vi "Tuning.vi"() -> ()   [LabVIEW 2018]
uses:
  Type/_GUI Method.ctl
  Type/_Lens Property.ctl
  Type/_Mass Range Property.ctl
  Type/_Mass Range Parameters.ctl
  Type/_RT Res Type.ctl
  Type/_Run Mode.ctl
  Type/_Run State.ctl
  Type/_File Type.ctl
  Type/_RT Command.ctl
  Type/_Data Operation.ctl
  Type/_Run Module.ctl
  Configuration/_Global Configuration.vi
  <vilib>/Utility/config.llb/Read Key (Path).vi
  <vilib>/Utility/config.llb/Read Key (Boolean).vi
  <vilib>/Utility/config.llb/Read Key (String).vi
  <vilib>/printing/ReportDocExtensions.llb/Append Front Panel Image to Report (path).vi
  <vilib>/Utility/config.llb/Write Key (Path).vi
  <vilib>/Utility/config.llb/Write Key (Boolean).vi
  <vilib>/Utility/config.llb/Write Key (String).vi
  <vilib>/Utility/miscctls.llb/LVRectTypeDef.ctl
  Type/_PIC Channel.ctl
  <vilib>/Utility/NIReport.llb/NI_report.lvclass
  <vilib>/Utility/NIReport.llb/NI_ReportGenerationCore.lvlib
  <vilib>/Utility/config.llb/NI_LVConfig.lvlib
panel:
  in  "Run 2":bool
  in  "Cancel":bool
  in  "NewMethod":bool
  in  "Method Path":path=path "C:/Users/Min/Projects/Sniffer/Build/Tune Method.d2m"
  in  "Tab":T1(tab)=enum."Mass Ranges"
  in  "Export Settings":bool
  out "Use Pol Swap Options from Config":bool
  in  "Delay Time (ms)":dbl=1.0 format="%#.3f"
  in  "CEM POL":bool
  in  "Polarity":enum32{"Positive Ions", "Negative Ions"}(radio) caption="Cal/Res Table Select"
  in  "Count1":dbl=420.0 caption="User Value" format="%.3f"
  in  "Q1DC POL":bool
  in  "Q2DC POL":bool
  out "DAC Value":i32=6174
  in  "Parameter Table":i32(listbox)
  in  "Swtich Polarity":bool
  in  "Ramping Parameter":u8(ring)=7 items=["Q1 RF", "Q1 DC", "Q1 RR", "Q2 RF", "Q2 DC", "Q2 RR", "M1 RF", "EV", "ED", "MO", "RO L1", "M1", "RO L2", "M2", "RO L3", "RO PF", "Q1", "CC L1", "CC L2", "CC", "CC L3", "CC L4", "Q2", "DD", "DISC", "DV", "DET horn", "HED", "EL", "LS400A", "LS-400A", "LS400B", "LS-400B", "QPS800", "QPS-800", "DG", "NG1", "HG1", "NG2", "HG2", "CC P", "SX", "ISV2", "ISV1", "CD", "CAP"]
  in  "Step Value":dbl=5.0 format="%#.3f"
  in  "Stop Value":dbl=80.0 format="%#.3f"
  in  "Start Value":dbl=10.0 format="%#.3f"
  in  "Perform Parameter Ramp":bool
  in  "Center/Width":bool
  in  "Scan Parameter with Mass":bool
  out "# of Steps":i32=141
  in  "Fixed Mass (amu)":dbl min=0.0
  in  "Scan Type":T2=enum."Q1 Scan"
  in  "Run Duration (s)":dbl=0.707 format="%#.3f"
  out "Cycle Time (ms)":dbl=706.0 format="%#.3f"
  in  "# of Cycles":i32=1
  in  "Pause Time (ms)":dbl=1.0 format="%#.3f"
  in  "Insert Row":bool
  in  "Delete Row":bool
  out "Ramp Time (ms)":dbl=705.0 format="%#.3f"
  in  "Dwell Time (ms)":dbl=5.0 min=0.001 format="%#.3f"
  in  "Step Mass (amu)":dbl=0.1 format="%#.3f"
  in  "Stop Mass (amu)":dbl=614.0 min=0.0 format="%#.3f"
  in  "Mass Range":i32(listbox)
  in  "Start Mass (amu)":dbl=600.0 min=0.0 format="%#.3f"
  in  "MR Parameters":bool
  in  "Resolution (Q1/Q2)":T3=2 items=["High/High", "Medium/Medium", "Low/Low", "High/Medium", "High/Low", "Medium/High", "Medium/Low", "Low/High", "Low/Medium"]
  in  "Method":T4={"Lenses"=[{"Scan Type"=0, "Scans"=1, "Time 1"=1.0, "Time 2"=1.0, "Value 1"=400.0, "Value 2"=400.0, "Step Size"=1.0}, {"Scan Type"=0, "Scans"=1, "Time 1"=1.0, "Time 2"=1.0, "Value 1"=150.0, "Value 2"=150.0, "Step Size"=1.0}, {"Scan Type"=0, "Scans"=1, "Time 1"=1.0, "Time 2"=1.0, "Value 1"=32000.0, "Value 2"=32000.0, "Step Size"=1.0}, {"Scan Type"=0, "Scans"=1, "Time 1"=1.0, "Time 2"=1.0, "Value 1"=400.0, "Value 2"=400.0, "Step Size"=1.0}, {"Scan Type"=0, "Scans"=1, "Time 1"=1.0, "Time 2"=1.0, "Value 1"=150.0, "Value 2"=150.0, "Step Size"=1.0}, {"Scan Type"=0, "Scans"=1, "Time 1"=1.0, "Time 2"=1.0, "Value 1"=64000.0, "Value 2"=64000.0, "Step Size"=1.0}, {"Scan Type"=0, "Scans"=1, "Time 1"=1.0, "Time 2"=1.0, "Value 1"=420.0, "Value 2"=420.0, "Step Size"=1.0}, {"Scan Type"=0, "Scans"=1, "Time 1"=1.0, "Time 2"=1.0, "Value 1"=30.0, "Value 2"=30.0, "Step Size"=1.0}, {"Scan Type"=0, "Scans"=1, "Time 1"=1.0, "Time 2"=1.0, "Value 1"=15.0, "Value 2"=15.0, "Step Size"=1.0}, {"Scan Type"=0, "Scans"=1, "Time 1"=1.0, "Time 2"=1.0, "Value 1"=0.0, "Value 2"=0.0, "Step Size"=1.0}, {"Scan Type"=0, "Scans"=1, "Time 1"=1.0, "Time 2"=1.0, "Value 1"=0.0, "Value 2"=0.0, "Step Size"=1.0}, {"Scan Type"=0, "Scans"=1, "Time 1"=1.0, "Time 2"=1.0, "Value 1"=0.0, "Value 2"=0.0, "Step Size"=1.0}, {"Scan Type"=0, "Scans"=1, "Time 1"=1.0, "Time 2"=1.0, "Value 1"=0.0, "Value 2"=0.0, "Step Size"=1.0}, {"Scan Type"=0, "Scans"=1, "Time 1"=1.0, "Time 2"=1.0, "Value 1"=0.0, "Value 2"=0.0, "Step Size"=1.0}, {"Scan Type"=0, "Scans"=1, "Time 1"=1.0, "Time 2"=1.0, "Value 1"=-0.5, "Value 2"=-0.5, "Step Size"=1.0}, {"Scan Type"=0, "Scans"=1, "Time 1"=1.0, "Time 2"=1.0, "Value 1"=-2.0, "Value 2"=-2.0, "Step Size"=1.0}, {"Scan Type"=0, "Scans"=1, "Time 1"=1.0, "Time 2"=1.0, "Value 1"=-1.2, "Value 2"=-1.2, "Step Size"=1.0}, {"Scan Type"=0, "Scans"=1, "Time 1"=1.0, "Time 2"=1.0, "Value 1"=0.0, "Value 2"=0.0, "Step Size"=1.0}, {"Scan Type"=0, "Scans"=1, "Time 1"=1.0, "Time 2"=1.0, "Value 1"=-240.0, "Value 2"=-240.0, "Step Size"=1.0}, {"Scan Type"=0, "Scans"=1, "Time 1"=1.0, "Time 2"=1.0, "Value 1"=-50.0, "Value 2"=-50.0, "Step Size"=1.0}, {"Scan Type"=0, "Scans"=1, "Time 1"=1.0, "Time 2"=1.0, "Value 1"=-52.0, "Value 2"=-52.0, "Step Size"=1.0}, {"Scan Type"=0, "Scans"=1, "Time 1"=1.0, "Time 2"=1.0, "Value 1"=-100.0, "Value 2"=-100.0, "Step Size"=1.0}, {"Scan Type"=0, "Scans"=1, "Time 1"=1.0, "Time 2"=1.0, "Value 1"=-54.0, "Value 2"=-54.0, "Step Size"=1.0}, {"Scan Type"=0, "Scans"=1, "Time 1"=1.0, "Time 2"=1.0, "Value 1"=-400.0, "Value 2"=-400.0, "Step Size"=1.0}, {"Scan Type"=0, "Scans"=1, "Time 1"=1.0, "Time 2"=1.0, "Value 1"=30.0, "Value 2"=30.0, "Step Size"=1.0}, {"Scan Type"=0, "Scans"=1, "Time 1"=1.0, "Time 2"=1.0, "Value 1"=2000.0, "Value 2"=2000.0, "Step Size"=1.0}, {"Scan Type"=0, "Scans"=1, "Time 1"=1.0, "Time 2"=1.0, "Value 1"=-6000.0, "Value 2"=-6000.0, "Step Size"=1.0}, {"Scan Type"=0, "Scans"=1, "Time 1"=1.0, "Time 2"=1.0, "Value 1"=0.0, "Value 2"=0.0, "Step Size"=1.0}, {"Scan Type"=0, "Scans"=1, "Time 1"=1.0, "Time 2"=1.0, "Value 1"=0.0, "Value 2"=0.0, "Step Size"=1.0}, {"Scan Type"=0, "Scans"=1, "Time 1"=1.0, "Time 2"=1.0, "Value 1"=250.0, "Value 2"=250.0, "Step Size"=1.0}, {"Scan Type"=0, "Scans"=1, "Time 1"=1.0, "Time 2"=1.0, "Value 1"=-250.0, "Value 2"=-250.0, "Step Size"=1.0}, {"Scan Type"=0, "Scans"=1, "Time 1"=1.0, "Time 2"=1.0, "Value 1"=250.0, "Value 2"=250.0, "Step Size"=1.0}, {"Scan Type"=0, "Scans"=1, "Time 1"=1.0, "Time 2"=1.0, "Value 1"=-250.0, "Value 2"=-250.0, "Step Size"=1.0}, {"Scan Type"=0, "Scans"=1, "Time 1"=1.0, "Time 2"=1.0, "Value 1"=500.0, "Value 2"=500.0, "Step Size"=1.0}, {"Scan Type"=0, "Scans"=1, "Time 1"=1.0, "Time 2"=1.0, "Value 1"=-500.0, "Value 2"=-500.0, "Step Size"=1.0}, {"Scan Type"=0, "Scans"=1, "Time 1"=1.0, "Time 2"=1.0, "Value 1"=0.55, "Value 2"=0.55, "Step Size"=1.0}, {"Scan Type"=0, "Scans"=1, "Time 1"=1.0, "Time 2"=1.0, "Value 1"=0.0, "Value 2"=0.0, "Step Size"=1.0}, {"Scan Type"=0, "Scans"=1, "Time 1"=1.0, "Time 2"=1.0, "Value 1"=100.0, "Value 2"=100.0, "Step Size"=1.0}, {"Scan Type"=0, "Scans"=1, "Time 1"=1.0, "Time 2"=1.0, "Value 1"=0.0, "Value 2"=0.0, "Step Size"=1.0}, {"Scan Type"=0, "Scans"=1, "Time 1"=1.0, "Time 2"=1.0, "Value 1"=5.0, "Value 2"=5.0, "Step Size"=1.0}, {"Scan Type"=0, "Scans"=1, "Time 1"=1.0, "Time 2"=1.0, "Value 1"=0.0, "Value 2"=0.0, "Step Size"=1.0}, {"Scan Type"=0, "Scans"=1, "Time 1"=1.0, "Time 2"=1.0, "Value 1"=0.0, "Value 2"=0.0, "Step Size"=1.0}, {"Scan Type"=0, "Scans"=1, "Time 1"=1.0, "Time 2"=1.0, "Value 1"=100.0, "Value 2"=100.0, "Step Size"=1.0}, {"Scan Type"=0, "Scans"=1, "Time 1"=1.0, "Time 2"=1.0, "Value 1"=0.0, "Value 2"=0.0, "Step Size"=1.0}, {"Scan Type"=0, "Scans"=1, "Time 1"=1.0, "Time 2"=1.0, "Value 1"=5.0, "Value 2"=5.0, "Step Size"=1.0}, {"Scan Type"=0, "Scans"=1, "Time 1"=1.0, "Time 2"=1.0, "Value 1"=5000.0, "Value 2"=5000.0, "Step Size"=1.0}, {"Scan Type"=0, "Scans"=1, "Time 1"=1.0, "Time 2"=1.0, "Value 1"=0.0, "Value 2"=0.0, "Step Size"=1.0}, {"Scan Type"=0, "Scans"=1, "Time 1"=1.0, "Time 2"=1.0, "Value 1"=100.0, "Value 2"=100.0, "Step Size"=1.0}, {"Scan Type"=0, "Scans"=1, "Time 1"=1.0, "Time 2"=1.0, "Value 1"=0.0, "Value 2"=0.0, "Step Size"=1.0}, {"Scan Type"=0, "Scans"=1, "Time 1"=1.0, "Time 2"=1.0, "Value 1"=5.0, "Value 2"=5.0, "Step Size"=1.0}, {"Scan Type"=0, "Scans"=1, "Time 1"=1.0, "Time 2"=1.0, "Value 1"=1000.0, "Value 2"=1000.0, "Step Size"=1.0}, {"Scan Type"=0, "Scans"=1, "Time 1"=1.0, "Time 2"=1.0, "Value 1"=1.0, "Value 2"=1.0, "Step Size"=1.0}], "Mass Ranges"=[{"Start"=600.0, "Stop"=614.0, "Step Size"=0.1, "Steps"=141, "Dwell"=5.0, "Parameters"=[], "Res"=2}], "Acquire"=FALSE, "MCA"=FALSE, "Q1DC EN"=FALSE, "Q1 POL"=FALSE, "Q3 POL"=FALSE, "Q1 RF  EN"=TRUE, "Averaging"=FALSE, "Log Scale"=FALSE, "CPS"=TRUE, "Unit"=FALSE, "Data Path"=path "C:/Users/Min/Projects/Sniffer/Build/My Data.isd", "Run Mode"=enum."Q1 Scan", "Fixed Mass (amu)"=0.0, "Q3DC EN"=FALSE, "Q3 RF  EN"=TRUE, "Negative"=FALSE} {"Mass Ranges"."Res" items=["High/High", "Medium/Medium", "Low/Low", "High/Medium", "High/Low", "Medium/High", "Medium/Low", "Low/High", "Low/Medium"]}
  out "Run Time":i32 caption="Run Time (ms)"
  in  "Log Scale":bool
  in  "Scan#":u32 caption="Current Scan #"
  in  "CPS":bool=TRUE
  in  "Averaging":bool
  in  "MCA":bool
  in  "Acquire":bool
  out "Spectrum":cluster{"Mass":dbl[], "Data in cps":dbl[]}[](graph)=[{"Mass"=[664.0], "Data in cps"=[]}, {"Mass"=[800.0], "Data in cps"=[]}, {"Mass"=[700.0], "Data in cps"=[]}]
  in  "BloUpdate":bool
  out "Data File:":path=path "C:/Users/Min/Projects/Sniffer/Build/My Data.isd"
  # "Selected Parameter Value"
  # "Selected Mass Range"
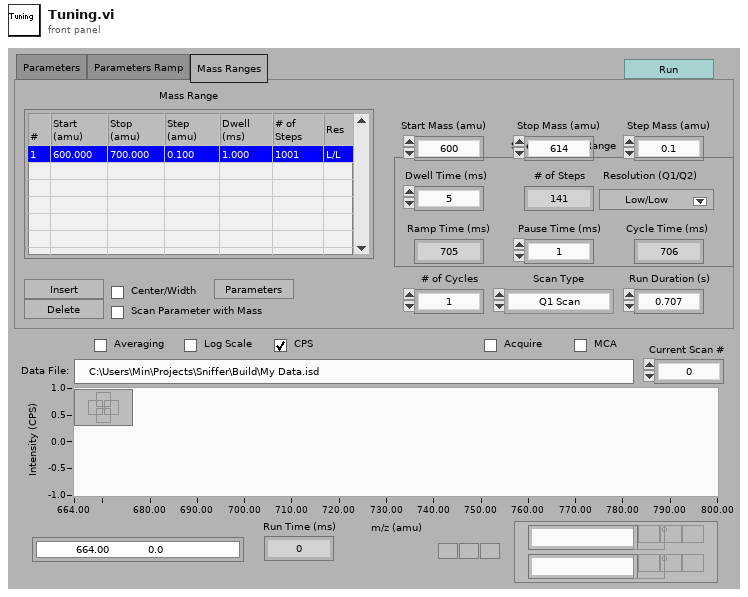
[diagram p1: front panel]
types:
  T1 = enum32{"Parameters", "Parameters Ramp", "Mass Ranges"}
  T2 = typedef "_Run Mode.ctl" = enum16{"MRM (Q1/Q2)", "Q1 Scan", "Q1 SRM", "Q2 Scan", "Q2 SRM", "Product Scan", "Precursor Scan", "Neutral Loss", "Neutral Gain"}
  T3 = typedef "_RT Res Type.ctl" = u16
  T4 = typedef "_GUI Method.ctl" = cluster{"Lenses":T5[], "Mass Ranges":T6[], "Acquire":bool, "MCA":bool, "Q1DC EN":bool, "Q1 POL":bool, "Q3 POL":bool, "Q1 RF  EN":bool, "Averaging":bool, "Log Scale":bool, "CPS":bool, "Unit":bool, "Data Path":path, "Run Mode":T2, "Fixed Mass (amu)":dbl, "Q3DC EN":bool, "Q3 RF  EN":bool, "Negative":bool}
  T5 = typedef "_Lens Property.ctl" = cluster{"Scan Type":u8, "Scans":i32, "Time 1":dbl, "Time 2":dbl, "Value 1":dbl, "Value 2":dbl, "Step Size":dbl}
  T6 = typedef "_Mass Range Property.ctl" = cluster{"Start":dbl, "Stop":dbl, "Step Size":dbl, "Steps":i32, "Dwell":dbl, "Parameters":T7[], "Res":T3}
  T7 = typedef "_Mass Range Parameters.ctl" = cluster{"Name":string, "Ch#":u8, "StartV":dbl, "StopV":dbl, "StepV":dbl, "Index":u8}
  T8 = typedef "_Run State.ctl" = enum16{"Init", "Update", "Start", "End", "Error"}
  T9 = typedef "_File Type.ctl" = enum16{"Configuration", "Old Configuration", "Calibration", "Resolution", "Diagnostic Method", "Old Method", "Acq Method", "Samp List"}
  T10 = typedef "LVRectTypeDef.ctl" = cluster{"Left":i16, "Top":i16, "Right":i16, "Bottom":i16}
  T11 = enum16{"Standard Report", "HTML", "Word", "Excel"}
  T12 = typedef "_RT Command.ctl" = enum16{"xml Start Run", "xml Start Actual Run", "xml Stop Run", "xml Runtime Update", "xml Get Status", "xml Get Table", "xml Set Table", "xml Get Configuration", "xml System Status", "xml Set LC Input Logic", "xml Get Data", "xml Get Info", "Start", "StartActualRun", "Stop", "Runtime Update", "Get Data", "Get Info", "Get Status", "Get Param", "Get Config", "Get Table", "Read ADC", "Set Oscillator", "Update Config", "Update Table", "Set All Pol", "Set Pol and DC", "Set Max Mass", "Toggle RP", "Toggle EL", "Set PIC", "Initialize Turbo", "Send Turbo Comm", "Close Turbo", "P1", "P2", "P3", "Send Serial", "Set LC Out", "Get LC In", "Read VAC", "Test Table", "Toggle Power", "Get Startup", "Set Startup", "Get ADC Table", "Set ADC Table", "Get Brief Status", "Get Detail Status", "Auxiliary Update", "Set CC Logics", "Set CC Input Logics", "Ignore Error", "invalid"}
  T13 = typedef "_Data Operation.ctl" = enum8{"Initialize", "Get Data", "Set Data", "Close"}
  T14 = enum32{"Bad", "Idle", "Run top level", "Running"}
  T15 = enum32{"existing file", "new file", "new or existing file", "existing dir", "new dir", "new or existing dir", "existing file (use LLBs)", "new file (use LLBs)", "new or existing file (use LLBs)", "new or existing file or directory (use LLBs)"}
  T16 = typedef "_PIC Channel.ctl" = enum16{"Corona +HV", "Corona -HV", "HSID Temp", "Time Const 1", "Curtain Cap +HV", "Curtain Cap -HV", "Time Const 2", "Source 1 +HV", "Source 1 -HV", "Source 1 Temp", "Time Const 3", "Source 2 +HV", "Source 2 -HV", "Source 2 Temp", "Time Const 4"}
  T17 = typedef "NI_LVConfig.lvlib/Config Data RefNum.ctl" = refnum<k1>
  T18 = typedef "_RT Instrument 2.ctl" = cluster{"Table":T19[], "Instrument":string[]}
  T19 = typedef "_RT Configuration 2.ctl" = cluster{"Name":string, "Ch#":u8, "Min":dbl, "Max":dbl, "Def+":dbl, "Def-":dbl, "Offset":dbl, "Slope":dbl, "Type":u8, "Description":string, "SettleT":dbl}
  T20 = cluster{"Method":T4, "Update":bool, "Running":bool, "Method Path":path, "BlockUpdate":bool}
  T21 = typedef "_Current Data.ctl" = cluster{"Scan#":i32, "Run Time (mS)":i32, "TIC X":dbl[], "TIC Y":dbl[][], "MassRange":cluster{"X Title":string, "X":dbl[], "Y":i32[]}[], "Fixed Mass (amu)":dbl, "Method":T22}
  T22 = typedef "_XML Expt.ctl" = cluster{"StartT(mS)":i32, "#Cycles":i32, "PauseT(uS)":i32, "ScanType":i32, "Polarity":u8, "FixedMass":dbl, "DelayT(mS)":i32, "Active Ch":T23[], "Mass Range":T6[]}
  T23 = typedef "_XML Lens.ctl" = cluster{"Value":dbl, "ChID":u8}
  T24 = typedef "_Run Module.ctl" = u16
  T25 = cluster{"Lenses":T5[], "Mass Ranges":T6[], "Acquire":bool, "MCA":bool, "Q1DC EN":bool, "Q1 POL":bool, "Q3 POL":bool, "Q1 RF  EN":bool, "Averaging":bool, "Log Scale":bool, "CPS":bool, "Unit":bool, "Data Path":path, "Run Mode":T2, "Fixed Mass (amu)":dbl, "Q3DC EN":bool, "Q3 RF  EN":bool, "Negative":bool}
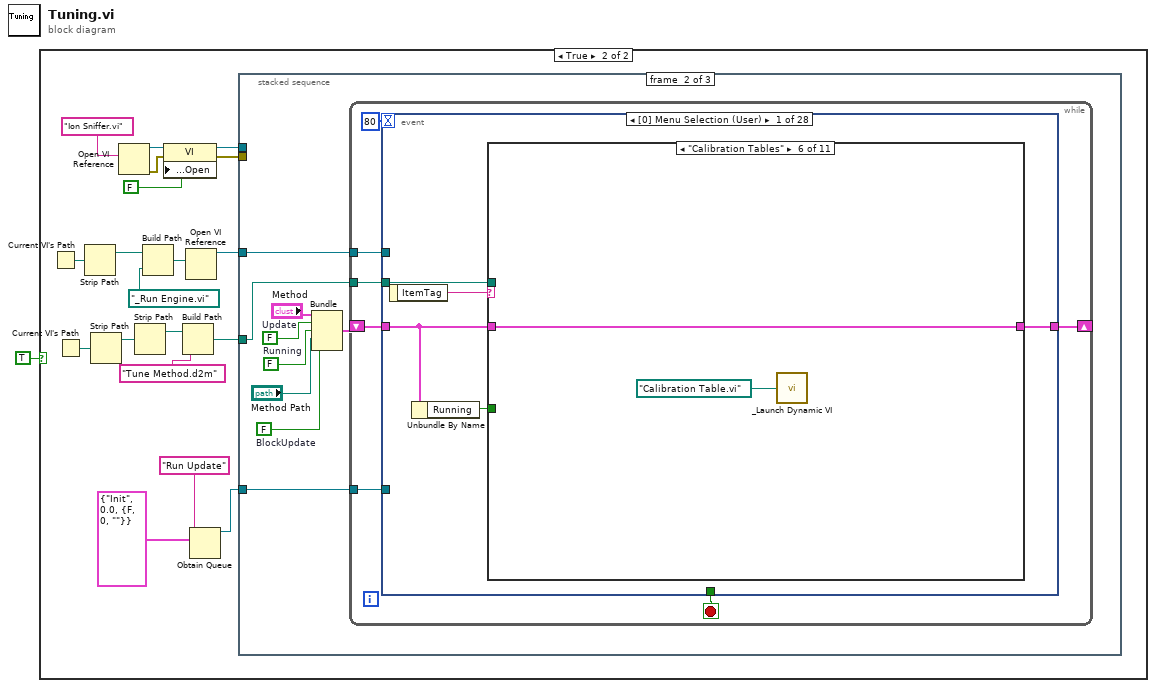
[diagram p0: block diagram]
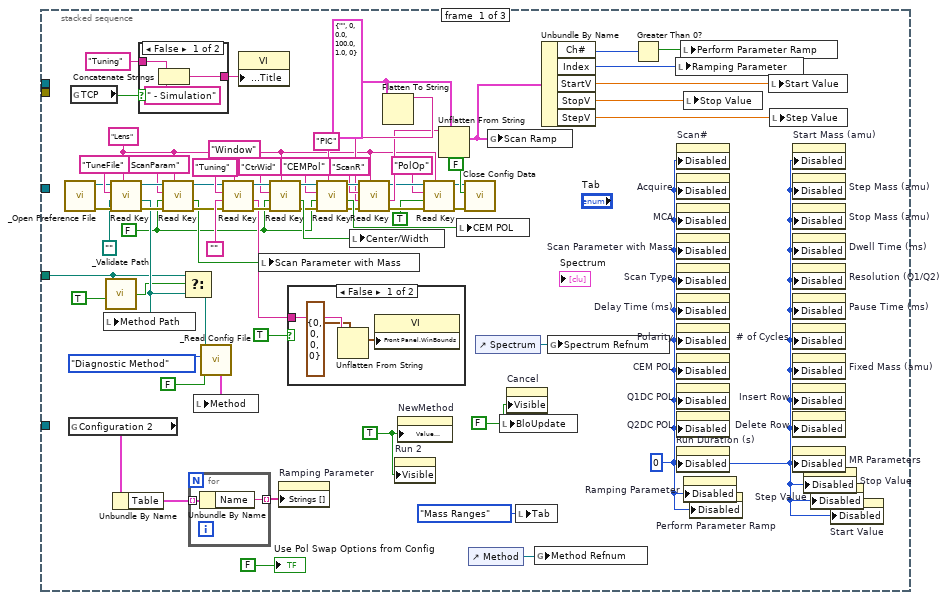
[diagram p3: hidden frame]
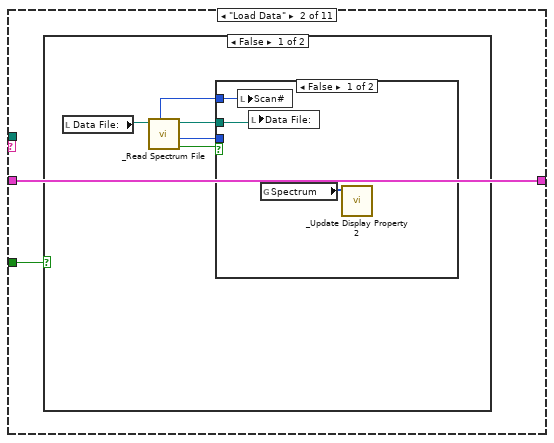
[diagram p7: hidden frame]
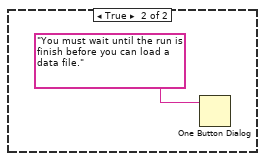
[diagram p9: hidden frame]
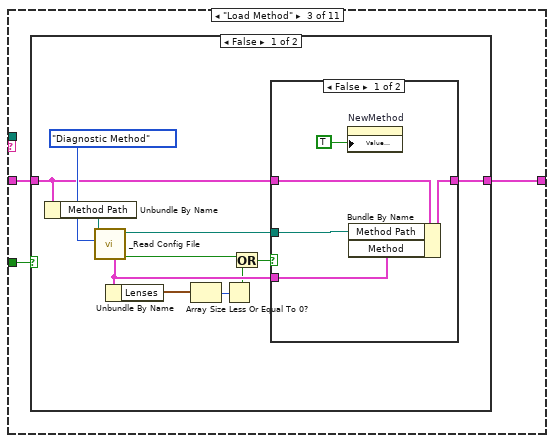
[diagram p10: hidden frame]
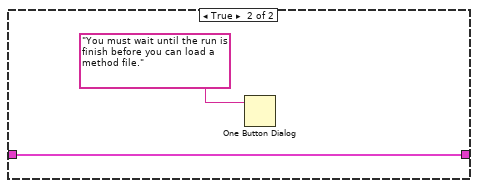
[diagram p12: hidden frame]
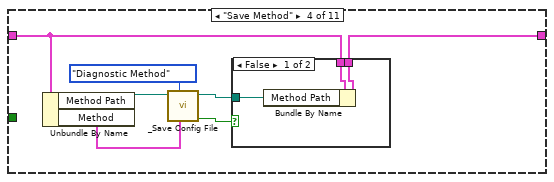
[diagram p13: hidden frame]
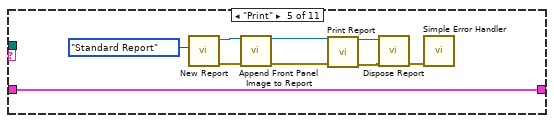
[diagram p15: hidden frame]
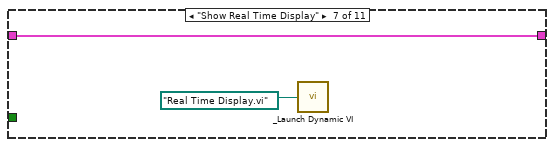
[diagram p16: hidden frame]
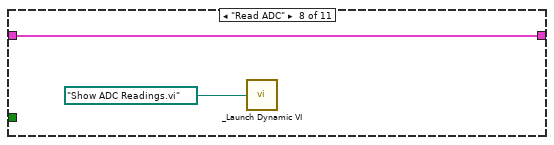
[diagram p17: hidden frame]
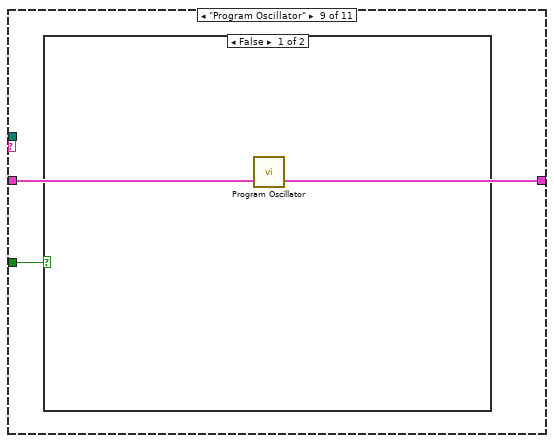
[diagram p18: hidden frame]
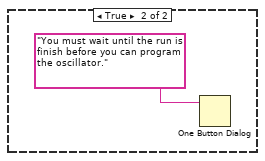
[diagram p19: hidden frame]
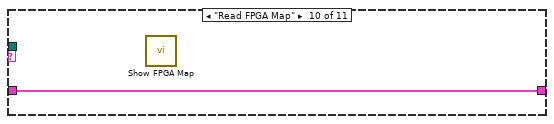
[diagram p20: hidden frame]
diagram:
  n1 = case shown="True" TRUE {
    frame False {
    }
    frame True {
      n2 = Current VI's Path() -> (path=w17:path)
      n3 = Current VI's Path() -> (path=w9:path)
      n4 = Strip Path(path=w17) -> (stripped path=w13:path)  [unwired: 1 out]
      n5 = Strip Path(path=w9) -> (stripped path=w10:path)  [unwired: 1 out]
      n6 = Open VI Reference(vi path="Ion Sniffer.vi") -> (vi reference=w5:refnum<vi>, error out=w6:errorcluster)  [unwired: 1 in, 4 out]
      n7 = Strip Path(path=w10) -> (stripped path=w11:path)  [unwired: 1 out]
      n8 = Build Path(base path=w13, name or relative path=path "_Run Engine.vi") -> (appended path=w15:path)
      n9 = property class="VI"(reference=w5, error in=w6, "Front Panel Window:Open"=FALSE) -> (reference out=w3:refnum<vi>, error out=w2:errorcluster)
      n10 = Build Path(base path=w11, name or relative path="Tune Method.d2m") -> (appended path=w8:path)
      n11 = Open VI Reference(vi path=w15) -> (vi reference=w14:refnum<vi>)  [unwired: 1 in, 5 out]
      n12 = Obtain Queue(name (unnamed)="Run Update", element data type=cluster{T8, dbl, "error out":errorcluster} {enum."Init", 0.0, "error out"={"status"=FALSE, "code"=0, "source"=""}}) -> (queue out=w18:refnum<queue>)  [unwired: 3 in, 2 out]
      n13 = stacked-sequence {
        tunnel: w18 -> [_ w105 w843]
        tunnel: w14 -> [_ w104 w842]
        tunnel: w8 -> [w50 w98 _]
        tunnel: w3 -> [_ _ w838]
        tunnel: w2 -> [_ _ w837]
        frame #0 {
          w42 = T7 {"Name"="", "Ch#"=0, "StartV"=0.0, "StopV"=100.0, "StepV"=1.0, "Index"=0} ("MR Parameters")
          w30 = u8 0 ("Disabled")
          w53 = FALSE
          w25 = "Lens" ("section")
          w71 = TRUE ("Visible")
          w79 = FALSE ("Unit")
          n14 = call "_Open Preference File.vi"() -> ("error"=w81:errorcluster, "refnum"=w82:T17)  [unwired: 3 in, 3 out]
          n15 = global read "_Global Configuration.vi" "Configuration 2"() -> (w35:T18)
          n16 = global read "_Global Configuration.vi" "TCP"() -> (w85:bool)
          n17 = call "_Validate Path.vi"("Check Exist (F)"=TRUE, "path"=w50) -> ("Valid"=w49:bool)  [unwired: 2 in]
          n18 = call-poly <vilib>:"Read Key.vi"("section"=w25, "error in (no error)"=w81, "default value"=path "", "key"="TuneFile", "refnum"=w82) -> ("error out"=w69:errorcluster, "value"=w68:path, "refnum out"=w67:T17)  [unwired: 4 out]
          n19 = local write "Method Path"(w68) -> ()
          n20 = Unbundle By Name(w35) -> ("Table"=w34:T19[])
          n21 = case shown="False" w85 {
            tunnel: "Tuning" ("string") -> [w95 w96]
            tunnel: [w93 w96] -> w86
            frame False {
              n22 = Concatenate Strings(w95, " - Simulation" ("string")) -> (w93:string)
            }
            frame True {
            }
          }
          n23 = call-poly <vilib>:"Read Key.vi"("section"=w25, "error in (no error)"=w69, "default value"=w53, "key"="ScanParam", "refnum"=w67) -> ("error out"=w64:errorcluster, "value"=w63:bool, "refnum out"=w65:T17)  [unwired: 4 out]
          n24 = Select(t=w50, s=w49, f=w68) -> (s? t:f=w75:path)
          n25 = for {
            tunnel: w34 -> [w89] mode=indexing
            tunnel: [w88] -> w33 mode=indexing
            n26 = Unbundle By Name(w89) -> ("Name"=w88:string)
          }
          n27 = call "_Read Config File.vi"("advisory dialog? (display:T)"=FALSE, "File Type (config)"=_File_Type."Diagnostic Method", "start path  (Not A Path)"=w75) -> ("GUI Method"=w77:T4)  [unwired: 8 out]
          n28 = local write "Method"(w77) -> ()
          n29 = call-poly <vilib>:"Read Key.vi"("section"="Window", "error in (no error)"=w64, "default value"="", "key"="Tuning" ("section"), "refnum"=w65) -> ("error out"=w62:errorcluster, "value"=w61:string, "refnum out"=w60:T17)  [unwired: 1 in, 3 out]
          n30 = property class="VI"("Front Panel Window:Title"=w86) -> ()  [unwired: 2 in, 2 out]
          n31 = local write "Scan Parameter with Mass"(w63) -> ()
          n32 = call-poly <vilib>:"Read Key.vi"("section"=w25, "error in (no error)"=w62, "default value"=w53, "key"="CtrWid", "refnum"=w60) -> ("error out"=w56:errorcluster, "value"=w58:bool, "refnum out"=w57:T17)  [unwired: 4 out]
          n33 = property on="Ramping Parameter" class="Ring (strict)"("Strings []"=w33) -> ()  [unwired: 2 in, 2 out]
          n34 = case shown="False" TRUE {
            tunnel: w61 -> [w92 _]
            frame False {
              n35 = Unflatten From String(type=T10 {"Left"=0, "Top"=0, "Right"=0, "Bottom"=0} ("Front Panel Window:Window Bounds"), binary string=w92) -> (value=w90:T10)  [unwired: 1 in, 4 out]
              n36 = property class="VI"("Front Panel.WinBounds"=w90) -> ()  [unwired: 2 in, 2 out]
            }
            frame True {
            }
          }
          n37 = call-poly <vilib>:"Read Key.vi"("section"="PIC", "error in (no error)"=w56, "default value"=w53, "key"="CEMPol" ("section"), "refnum"=w57) -> ("error out"=w46:errorcluster, "value"=w52:bool, "refnum out"=w47:T17)  [unwired: 4 out]
          n38 = local write "Center/Width"(w58) -> ()
          n39 = Flatten To String(anything=w42) -> (data string=w43:string)  [unwired: 1 in, 4 out]
          n40 = call-poly <vilib>:"Read Key.vi"("section"=w25, "error in (no error)"=w46, "default value"=w43, "key"="ScanR" ("section"), "refnum"=w47) -> ("error out"=w26:errorcluster, "value"=w41:string, "refnum out"=w27:T17)  [unwired: 1 in, 3 out]
          n41 = property on="Run 2" class="Bool"("Visible"=w71) -> ()  [unwired: 2 in, 2 out]
          n42 = property on="NewMethod" class="Bool (strict)"("Value (Signaling)"=w71) -> ()  [unwired: 2 in, 2 out]
          n43 = call-poly <vilib>:"Read Key.vi"("section"=w25, "error in (no error)"=w26, "default value"=TRUE, "key"="PolOp" ("section"), "refnum"=w27) -> ("error out"=w29:errorcluster, "refnum out"=w28:T17)  [unwired: 5 out]
          n44 = Unflatten From String(type=w42, binary string=w41) -> (value=w40:T7)  [unwired: 1 in, 4 out]
          n45 = local write "CEM POL"(w52) -> ()
          n46 = call <vilib>:"Close Config Data.vi"("error in (no error)"=w29, "write file if changed (T)"=FALSE ("write configuration file? (F)"), "refnum"=w28) -> ()  [unwired: 9 out]
          n47 = control-ref of="Method"() -> (w44:refnum<vi>)
          n48 = control-ref of="Spectrum"() -> (w70:refnum<vi>)
          n49 = global write "_Global Configuration.vi" "Scan Ramp"(w40) -> ()
          n50 = local write "BloUpdate"(w79) -> ()
          n51 = property on="Cancel" class="Bool"("Visible"=w79) -> ()  [unwired: 2 in, 2 out]
          n52 = local write "Tab"(T1."Mass Ranges" ("Tab")) -> ()
          n53 = global write "_Global Configuration.vi" "Method Refnum"(w44) -> ()
          n54 = Unbundle By Name(w40) -> ("Ch#"=w32:u8, "Index"=w39:u8, "StartV"=w38:dbl, "StopV"=w37:dbl, "StepV"=w36:dbl)
          n55 = global write "_Global Configuration.vi" "Spectrum Refnum"(w70) -> ()
          n56 = Greater Than 0?(x=w32) -> (x > 0?=w31:bool)
          n57 = local write "Ramping Parameter"(w39) -> ()
          n58 = property on="Scan#" class="DigNum (strict)"("Disabled"=w30) -> ()  [unwired: 2 in, 2 out]
          n59 = property on="Acquire" class="Bool (strict)"("Disabled"=w30) -> ()  [unwired: 2 in, 2 out]
          n60 = property on="MCA" class="Bool (strict)"("Disabled"=w30) -> ()  [unwired: 2 in, 2 out]
          n61 = property on="Scan Parameter with Mass" class="Bool (strict)"("Disabled"=w30) -> ()  [unwired: 2 in, 2 out]
          n62 = property on="Scan Type" class="Enum (strict)"("Disabled"=w30) -> ()  [unwired: 2 in, 2 out]
          n63 = property on="Delay Time (ms)" class="DigNum (strict)"("Disabled"=w30) -> ()  [unwired: 2 in, 2 out]
          n64 = property on="Polarity" class="RadioBtnsControl (strict)"("Disabled"=w30) -> ()  [unwired: 2 in, 2 out]
          n65 = property on="CEM POL" class="Bool (strict)"("Disabled"=w30) -> ()  [unwired: 2 in, 2 out]
          n66 = property on="Q1DC POL" class="Bool (strict)"("Disabled"=w30) -> ()  [unwired: 2 in, 2 out]
          n67 = property on="Q2DC POL" class="Bool (strict)"("Disabled"=w30) -> ()  [unwired: 2 in, 2 out]
          n68 = property on="Run Duration (s)" class="DigNum (strict)"("Disabled"=w30) -> ()  [unwired: 2 in, 2 out]
          n69 = local write "Perform Parameter Ramp"(w31) -> ()
          n70 = local write "Stop Value"(w37) -> ()
          n71 = property on="Ramping Parameter" class="Ring (strict)"("Disabled"=w30) -> ()  [unwired: 2 in, 2 out]
          n72 = property on="Perform Parameter Ramp" class="Bool (strict)"("Disabled"=w30) -> ()  [unwired: 2 in, 2 out]
          n73 = local write "Start Value"(w38) -> ()
          n74 = local write "Step Value"(w36) -> ()
          n75 = property on="Start Mass (amu)" class="DigNum (strict)"("Disabled"=w30) -> ()  [unwired: 2 in, 2 out]
          n76 = property on="Step Mass (amu)" class="DigNum (strict)"("Disabled"=w30) -> ()  [unwired: 2 in, 2 out]
          n77 = property on="Stop Mass (amu)" class="DigNum (strict)"("Disabled"=w30) -> ()  [unwired: 2 in, 2 out]
          n78 = property on="Dwell Time (ms)" class="DigNum (strict)"("Disabled"=w30) -> ()  [unwired: 2 in, 2 out]
          n79 = property on="Resolution (Q1/Q2)" class="Ring (strict)"("Disabled"=w30) -> ()  [unwired: 2 in, 2 out]
          n80 = property on="Pause Time (ms)" class="DigNum (strict)"("Disabled"=w30) -> ()  [unwired: 2 in, 2 out]
          n81 = property on="# of Cycles" class="DigNum (strict)"("Disabled"=w30) -> ()  [unwired: 2 in, 2 out]
          n82 = property on="Fixed Mass (amu)" class="DigNum (strict)"("Disabled"=w30) -> ()  [unwired: 2 in, 2 out]
          n83 = property on="Insert Row" class="Bool"("Disabled"=w30) -> ()  [unwired: 2 in, 2 out]
          n84 = property on="Delete Row" class="Bool"("Disabled"=w30) -> ()  [unwired: 2 in, 2 out]
          n85 = property on="MR Parameters" class="Bool"("Disabled"=w30) -> ()  [unwired: 2 in, 2 out]
          n86 = property on="Stop Value" class="DigNum (strict)"("Disabled"=w30) -> ()  [unwired: 2 in, 2 out]
          n87 = property on="Step Value" class="DigNum (strict)"("Disabled"=w30) -> ()  [unwired: 2 in, 2 out]
          n88 = property on="Start Value" class="DigNum (strict)"("Disabled"=w30) -> ()  [unwired: 2 in, 2 out]
          "Use Pol Swap Options from Config" <- FALSE ("Use Pol Swap Options from Config")
        }
        frame #1 {
          w97 = FALSE  # BlockUpdate
          w101 = FALSE  # Running
          w102 = FALSE  # Update
          n89 = Bundle("Method"="Method", "Update"=w102, "Running"=w101, "Method Path"="Method Path", "BlockUpdate"=w97) -> (w100:T20)  [unwired: 1 out]
          n90 = while {
            shift-right: [w109] -> _
            shift-left: w100 -> [w111]
            tunnel: w105 -> [w108]
            tunnel: w104 -> [w107]
            tunnel: w98 -> [w106]
            stop <- w112 stop-if-true
            n91 = event shown="[0] Menu Selection (User)" {
              selector: _ -> [_ _ _ _ _ _ _ _ _ _ _ _ _ _ _ _ _ _ _ _ _ _ _ _ _ _ _ _]
              dyn-events: _ -> [_ _ _ _ _ _ _ _ _ _ _ _ _ _ _ _ _ _ _ _ _ _ _ _ _ _ _ _]
              timeout: 80 -> [_ _ _ _ _ _ _ _ _ _ _ _ _ _ _ _ _ _ _ _ _ _ _ _ _ _ _ _]
              tunnel: [_ w191 _ _ _ _ _ _ _ _ _ _ _ _ _ _ _ _ _ _ _ _ _ _ _ _ _ _] -> w112
              tunnel: w111 -> [w115 w220 w229 w294 w326 w356 w368 w393 w462 w477 w507 w541 w563 w576 w591 w596 w628 w678 w697 w727 w738 w751 w773 w777 w784 w801 w804 w836]
              tunnel: [w116 w220 w231 w293 w323 w355 w367 w392 w461 w477 w508 w542 w563 w575 w587 w598 w627 w678 w697 w726 w738 w744 w771 w776 w782 w796 w804 w836] -> w109
              tunnel: w108 -> [_ _ w230 _ w327 _ _ _ _ _ _ _ _ _ _ _ _ _ _ _ _ _ _ _ _ _ _ _]
              tunnel: w107 -> [_ _ _ _ w328 w354 _ _ _ _ _ _ _ _ _ _ _ _ _ _ _ _ _ _ _ _ _ _]
              tunnel: w106 -> [w113 w217 _ _ _ _ _ _ _ _ _ _ _ _ _ _ _ _ _ _ _ _ _ _ _ _ _ _]
              event Menu Selection (User) {
                n92 = event-data() -> ("ItemTag"=w117:string)  [unwired: 1 out]
                n93 = Unbundle By Name(w115) -> ("Running"=w114:bool)
                n94 = case shown="\"Calibration Tables\"" w117 {
                  tunnel: w114 -> [_ w120 w132 _ _ _ _ _ w179 _ _]
                  tunnel: w115 -> [w118 w119 w131 w153 w165 w172 w175 w176 w178 w181 w182]
                  tunnel: [w118 w119 w130 w152 w165 w172 w175 w176 w178 w181 w182] -> w116
                  tunnel: w113 -> [_ _ _ _ _ _ _ _ _ _ _]
                  frame Default {
                  }
                  frame "Load Data" {
                    n95 = case shown="False" w120 {
                      frame False {
                        n96 = local read "Data File:"() -> (w123:path)
                        n97 = call "_Read Spectrum File.vi"("start path  (Not A Path)"=w123) -> ("error"=w125:bool, "TIC"=w124:u32, "new file path"=w122:path, "Scan# out"=w121:u32)  [unwired: 2 in, 3 out]
                        n98 = case shown="False" w125 {
                          tunnel: w124 -> [_ _]
                          tunnel: w122 -> [w128 _]
                          tunnel: w121 -> [w127 _]
                          frame False {
                            n99 = local write "Scan#"(w127) -> ()
                            n100 = local write "Data File:"(w128) -> ()
                            n101 = global read "_Global Configuration.vi" "Spectrum"() -> (w126:i32[])
                            n102 = call "_Update Display Property 2.vi"("Spectrum in"=w126) -> ()  [unwired: 7 out]
                          }
                          frame True {
                          }
                        }
                      }
                      frame True {
                        n103 = One Button Dialog(message="You must wait until the run is finish before you can load a data file.") -> ()  [unwired: 2 out]
                      }
                    }
                  }
                  frame "Load Method" {
                    n104 = case shown="False" w132 {
                      tunnel: w131 -> [w141 w150]
                      tunnel: [w133 w150] -> w130
                      frame False {
                        n105 = Unbundle By Name(w141) -> ("Method Path"=w143:path)
                        n106 = call "_Read Config File.vi"("File Type (config)"=_File_Type."Diagnostic Method", "start path  (Not A Path)"=w143) -> ("error"=w136:bool, "new file path"=w140:path, "GUI Method"=w139:T4)  [unwired: 1 in, 6 out]
                        n107 = Unbundle By Name(w139) -> ("Lenses"=w138:T5[])
                        n108 = Array Size(array=w138) -> (size(s)=w137:i32)
                        n109 = Less Or Equal To 0?(x=w137) -> (x <= 0?=w135:bool)
                        n110 = Or(x=w136, y=w135) -> (x .or. y?=w134:bool)
                        n111 = case shown="False" w134 {
                          tunnel: w141 -> [w148 w149]
                          tunnel: w139 -> [w145 _]
                          tunnel: w140 -> [w146 _]
                          tunnel: [w147 w149] -> w133
                          frame False {
                            n112 = property on="NewMethod" class="Bool (strict)"("Value (Signaling)"=TRUE) -> ()  [unwired: 2 in, 2 out]
                            n113 = Bundle By Name(cluster=w148, "Method Path"=w146, "Method"=w145) -> (w147:T20)
                          }
                          frame True {
                          }
                        }
                      }
                      frame True {
                        n114 = One Button Dialog(message="You must wait until the run is finish before you can load a method file.") -> ()  [unwired: 2 out]
                      }
                    }
                  }
                  frame "Save Method" {
                    n115 = Unbundle By Name(w153) -> ("Method Path"=w156:path, "Method"=w154:T4)
                    n116 = call "_Save Config File.vi"("GUI Method"=w154, "File Type (config)"=_File_Type."Diagnostic Method", "start path  (Not A Path)"=w156) -> ("error"=w157:bool, "new file path"=w158:path)  [unwired: 5 in, 2 out]
                    n117 = case shown="False" w157 {
                      tunnel: w158 -> [w160 _]
                      tunnel: w153 -> [w161 w162]
                      tunnel: [w159 w162] -> w152
                      frame False {
                        n118 = Bundle By Name(cluster=w161, "Method Path"=w160) -> (w159:T20)
                      }
                      frame True {
                      }
                    }
                  }
                  frame "Print" {
                    n119 = call <vilib>:"New Report.vi"("report type"=T11."Standard Report") -> ("report out"=w169:refnum<class "NI_report.lvclass">, "error out"=w168:errorcluster)  [unwired: 5 in, 8 out]
                    n120 = call-poly <vilib>:"Append Front Panel Image to Report.vi"("report in"=w169, "error in (no error)"=w168) -> ("report out"=w167:refnum<class "NI_report.lvclass">, "error out"=w166:errorcluster)  [unwired: 6 in, 6 out]
                    n121 = call-dynamic "Print Report.vi"("report in"=w167, "error in (no error)"=w166) -> ("report out"=w171:refnum<class "NI_report.lvclass">, "error out"=w170:errorcluster)  [unwired: 2 in, 10 out]
                    n122 = call-dynamic "Dispose Report.vi"("report in"=w171, "error in (no error)"=w170) -> ("error out"=w164:errorcluster)  [unwired: 3 in, 10 out]
                    n123 = call <vilib>:"Simple Error Handler.vi"("error in (no error)"=w164) -> ()  [unwired: 1 in, 8 out]
                  }
                  frame "Calibration Tables" {
                    n124 = call "_Launch Dynamic VI.vi"("VI Name"=path "Calibration Table.vi" ("name or relative path")) -> ()  [unwired: 3 in, 1 out]
                  }
                  frame "Show Real Time Display" {
                    n125 = call "_Launch Dynamic VI.vi"("VI Name"=path "Real Time Display.vi" ("name or relative path")) -> ()  [unwired: 3 in, 1 out]
                  }
                  frame "Read ADC" {
                    n126 = call "_Launch Dynamic VI.vi"("VI Name"=path "Show ADC Readings.vi" ("name or relative path")) -> ()  [unwired: 3 in, 1 out]
                  }
                  frame "Program Oscillator" {
                    n127 = case shown="False" w179 {
                      frame False {
                        n128 = call "Program Oscillator.vi"() -> ()  [unwired: 1 out]
                      }
                      frame True {
                        n129 = One Button Dialog(message="You must wait until the run is finish before you can program the oscillator.") -> ()  [unwired: 2 out]
                      }
                    }
                  }
                  frame "Read FPGA Map" {
                    n130 = call "Show FPGA Map.vi"() -> ()  [unwired: 12 out]
                  }
                  frame "About" {
                    n131 = call "About Box.vi"() -> ()  [unwired: 1 out]
                  }
                }
              }
              event Panel Close? {
                w185 = "Lens" ("section")
                (unwired) TRUE
                w191 = TRUE ("Discard?")
                n132 = event-data() -> ()  [unwired: 4 out]
                n133 = Unbundle By Name(w220) -> ("Method Path"=w219:path, "Method"=w216:T4)
                n134 = global read "_Global Configuration.vi" "Scan Ramp"() -> (w190:T7)
                n135 = call "_Open Preference File.vi"() -> ("error"=w222:errorcluster, "refnum"=w223:T17)  [unwired: 3 in, 3 out]
                n136 = local read "Scan Parameter with Mass"() -> (w207:bool)
                n137 = property class="VI"() -> ("Front Panel.WinBounds"=w213:T10)  [unwired: 2 in, 2 out]
                n138 = call-poly <vilib>:"Write Key.vi"("section"=w185, "error in (no error)"=w222, "value"=w219, "key"="TuneFile", "refnum"=w223) -> ("error out"=w211:errorcluster, "refnum out"=w210:T17)  [unwired: 5 out]
                n139 = local read "Center/Width"() -> (w203:bool)
                n140 = call-poly <vilib>:"Write Key.vi"("section"=w185, "error in (no error)"=w211, "value"=w207, "key"="ScanParam", "refnum"=w210) -> ("error out"=w206:errorcluster, "refnum out"=w205:T17)  [unwired: 5 out]
                n141 = Flatten To String(anything=w213) -> (data string=w212:string)  [unwired: 1 in, 4 out]
                n142 = call-poly <vilib>:"Write Key.vi"("section"=w185, "error in (no error)"=w206, "value"=w203, "key"="CtrWid", "refnum"=w205) -> ("error out"=w201:errorcluster, "refnum out"=w202:T17)  [unwired: 5 out]
                n143 = local read "CEM POL"() -> (w196:bool)
                n144 = Flatten To String(anything=w190) -> (data string=w192:string)  [unwired: 1 in, 4 out]
                n145 = call-poly <vilib>:"Write Key.vi"("section"="Window", "error in (no error)"=w201, "value"=w212, "key"="Tuning" ("section"), "refnum"=w202) -> ("error out"=w200:errorcluster, "refnum out"=w199:T17)  [unwired: 1 in, 4 out]
                n146 = call-poly <vilib>:"Write Key.vi"("section"="PIC", "error in (no error)"=w200, "value"=w196, "key"="CEMPol" ("section"), "refnum"=w199) -> ("error out"=w195:errorcluster, "refnum out"=w194:T17)  [unwired: 5 out]
                n147 = call "_Save Config File.vi"("GUI Method"=w216, "File Type (config)"=_File_Type."Diagnostic Method", "advisory dialog? (display:T)"=FALSE, "start path  (Not A Path)"=w217) -> ()  [unwired: 4 in, 4 out]
                n148 = call-poly <vilib>:"Write Key.vi"("section"=w185, "error in (no error)"=w195, "value"=w192, "key"="ScanR" ("section"), "refnum"=w194) -> ("error out"=w186:errorcluster, "refnum out"=w187:T17)  [unwired: 1 in, 4 out]
                n149 = global write "_Global Configuration.vi" "Run"(FALSE ("Update")) -> ()
                n150 = call-poly <vilib>:"Write Key.vi"("section"=w185, "error in (no error)"=w186, "value"=FALSE, "key"="PolOp" ("section"), "refnum"=w187) -> ("error out"=w189:errorcluster, "refnum out"=w188:T17)  [unwired: 5 out]
                n151 = call <vilib>:"Close Config Data.vi"("error in (no error)"=w189, "write file if changed (T)"=TRUE ("write configuration file? (F)"), "refnum"=w188) -> ()  [unwired: 9 out]
                n152 = call "_Remote Communicate.vi"("Command"=_RT_Command."Stop") -> ()  [unwired: 5 in, 4 out]
                n153 = event-data("Discard?"=w191) -> ()  [unwired: 1 in, 1 out]
              }
              event Timeout {
                n154 = event-data() -> ()  [unwired: 4 out]
                n155 = Unbundle By Name(w229) -> ("Update"=w228:bool, "Running"=w227:bool)
                n156 = case shown="True" w228 {
                  tunnel: w229 -> [w241 w281]
                  tunnel: [w240 w279] -> w231
                  tunnel: w227 -> [w243 _]
                  tunnel: w230 -> [w242 _]
                  frame False {
                    n157 = local read "Scan#"() -> (w237:u32)
                    n158 = call "_Current Data Global.vi"("Operation"=_Data_Operation."Get Data") -> ("Latest Raw Data"=w238:i32[], "CurrentData"=w234:T21[])  [unwired: 3 in, 2 out]
                    n159 = case shown="True" w243 {
                      tunnel: w242 -> [_ w253]
                      tunnel: w241 -> [w247 w249]
                      tunnel: [w247 w248] -> w240
                      frame False {
                      }
                      frame True {
                        n160 = Dequeue Element(queue=w253, timeout in ms (-1)=1) -> (element=w251:cluster{T8, dbl, "error out":errorcluster}, timed out?=w250:bool)  [unwired: 1 in, 2 out]
                        n161 = case shown="False" w250 {
                          tunnel: w251 -> [w259 _]
                          tunnel: w249 -> [w255 w270]
                          tunnel: [w254 w270] -> w248
                          frame False {
                            n162 = Unbundle(w259) -> (w258:T8, w256:dbl, "error out"=w257:errorcluster)
                            n163 = case shown="\"End\"" w258 {
                              tunnel: w257 -> [_ w266 w269]
                              tunnel: w256 -> [_ _ _]
                              tunnel: w255 -> [w260 w265 w268]
                              tunnel: [w260 w264 w268] -> w254
                              frame "Init", Default {
                              }
                              frame "End" {
                                w261 = u8 0 ("Disabled")
                                n164 = property on="Scan#" class="DigNum (strict)"("Disabled"=w261) -> ()  [unwired: 2 in, 2 out]
                                n165 = property on="Acquire" class="Bool (strict)"("Disabled"=w261) -> ()  [unwired: 2 in, 2 out]
                                n166 = property on="MCA" class="Bool (strict)"("Disabled"=w261) -> ()  [unwired: 2 in, 2 out]
                                n167 = property on="Scan Parameter with Mass" class="Bool (strict)"("Disabled"=w261) -> ()  [unwired: 2 in, 2 out]
                                n168 = property on="Ramping Parameter" class="Ring (strict)"("Disabled"=w261) -> ()  [unwired: 2 in, 2 out]
                                n169 = property on="Scan Type" class="Enum (strict)"("Disabled"=w261) -> ()  [unwired: 2 in, 2 out]
                                n170 = property on="Perform Parameter Ramp" class="Bool (strict)"("Disabled"=w261) -> ()  [unwired: 2 in, 2 out]
                                n171 = property on="Delay Time (ms)" class="DigNum (strict)"("Disabled"=w261) -> ()  [unwired: 2 in, 2 out]
                                n172 = property on="Polarity" class="RadioBtnsControl (strict)"("Disabled"=w261) -> ()  [unwired: 2 in, 2 out]
                                n173 = property on="CEM POL" class="Bool (strict)"("Disabled"=w261) -> ()  [unwired: 2 in, 2 out]
                                n174 = property on="Q1DC POL" class="Bool (strict)"("Disabled"=w261) -> ()  [unwired: 2 in, 2 out]
                                n175 = property on="Q2DC POL" class="Bool (strict)"("Disabled"=w261) -> ()  [unwired: 2 in, 2 out]
                                n176 = property on="Run Duration (s)" class="DigNum (strict)"("Disabled"=w261) -> ()  [unwired: 2 in, 2 out]
                                n177 = property on="Start Mass (amu)" class="DigNum (strict)"("Disabled"=w261) -> ()  [unwired: 2 in, 2 out]
                                n178 = property on="Step Mass (amu)" class="DigNum (strict)"("Disabled"=w261) -> ()  [unwired: 2 in, 2 out]
                                n179 = property on="Stop Mass (amu)" class="DigNum (strict)"("Disabled"=w261) -> ()  [unwired: 2 in, 2 out]
                                n180 = property on="Dwell Time (ms)" class="DigNum (strict)"("Disabled"=w261) -> ()  [unwired: 2 in, 2 out]
                                n181 = property on="Resolution (Q1/Q2)" class="Ring (strict)"("Disabled"=w261) -> ()  [unwired: 2 in, 2 out]
                                n182 = property on="Pause Time (ms)" class="DigNum (strict)"("Disabled"=w261) -> ()  [unwired: 2 in, 2 out]
                                n183 = property on="# of Cycles" class="DigNum (strict)"("Disabled"=w261) -> ()  [unwired: 2 in, 2 out]
                                n184 = property on="Fixed Mass (amu)" class="DigNum (strict)"("Disabled"=w261) -> ()  [unwired: 2 in, 2 out]
                                n185 = property on="Insert Row" class="Bool"("Disabled"=w261) -> ()  [unwired: 2 in, 2 out]
                                n186 = property on="Delete Row" class="Bool"("Disabled"=w261) -> ()  [unwired: 2 in, 2 out]
                                n187 = property on="MR Parameters" class="Bool"("Disabled"=w261) -> ()  [unwired: 2 in, 2 out]
                                n188 = property on="Stop Value" class="DigNum (strict)"("Disabled"=w261) -> ()  [unwired: 2 in, 2 out]
                                n189 = property on="Step Value" class="DigNum (strict)"("Disabled"=w261) -> ()  [unwired: 2 in, 2 out]
                                n190 = property on="Start Value" class="DigNum (strict)"("Disabled"=w261) -> ()  [unwired: 2 in, 2 out]
                                n191 = Bundle By Name(cluster=w265, "Running"=FALSE) -> (w264:T20)
                                n192 = property on="Run 2" class="Bool"("Visible"=TRUE) -> ()  [unwired: 2 in, 2 out]
                                n193 = property on="Cancel" class="Bool"("Visible"=FALSE) -> ()  [unwired: 2 in, 2 out]
                                n194 = call "_Handle Error.vi"("error in (no error)"=w266) -> ()  [unwired: 2 in, 5 out]
                              }
                              frame "Error" {
                                n195 = call "_Handle Error.vi"("error in (no error)"=w269) -> ()  [unwired: 2 in, 5 out]
                              }
                            }
                          }
                          frame True {
                          }
                        }
                      }
                    }
                    n196 = Index Array(array=w234) -> (element=w233:T21)  [unwired: 1 in]
                    n197 = Unbundle By Name(w233) -> ("Scan#"=w232:i32, "Run Time (mS)"=w236:i32)
                    n198 = Not Equal?(x=w232, y=w237) -> (x != y?=w235:bool)
                    n199 = case shown="True" w235 {
                      tunnel: w232 -> [_ w246]
                      tunnel: w238 -> [_ w244]
                      tunnel: w236 -> [_ w245]
                      frame False {
                      }
                      frame True {
                        n200 = local write "Scan#"(w246) -> ()
                        n201 = global write "_Global Configuration.vi" "Spectrum"(w244) -> ()
                        n202 = call "_Update Display Property 2.vi"("Spectrum in"=w244) -> ()  [unwired: 7 out]
                        "Run Time" <- w245
                      }
                    }
                  }
                  frame True {
                    n203 = Unbundle By Name(w281) -> ("Method"=w282:T4)
                    n204 = property on="BloUpdate" class="Bool (strict)"("Value (Signaling)"=TRUE) -> ()  [unwired: 2 in, 2 out]
                    n205 = property on="Parameter Table" class="MCListbox (strict)"() -> ("Item Names"=w274:string[][])  [unwired: 2 in, 2 out]
                    n206 = Index Array(array=w274, index (row)="Parameter Table", index (col)=0 ("disabled index (col)")) -> (element=w276:string)
                    n207 = call "_Get Lens Configuration.vi"("Name"=w276) -> ("Found"=w271:bool, "Config Row#"=w272:i32)  [unwired: 1 in, 4 out]
                    n208 = case shown="True" w271 {
                      tunnel: w282 -> [w283 w289]
                      tunnel: [w283 w288] -> w278
                      tunnel: w272 -> [_ w287]
                      frame False {
                      }
                      frame True {
                        n209 = call "_Validate Tune Property.vi"("ConfigRow #"=w287, "User Value"="Count1", "Method In"=w289) -> ("Lens Table"=w290:string[][], "DAC Value Out"=→"DAC Value":i32, "User Value Out"=w285:dbl, "Method Out"=w288:T4)  [unwired: 2 out]
                        n210 = local write "Method"(w288) -> ()
                        n211 = property on="Parameter Table" class="MCListbox (strict)"("Item Names"=w290) -> ()  [unwired: 2 in, 2 out]
                        n212 = local write "Count1"(w285) -> ()
                      }
                    }
                    n213 = Bundle By Name(cluster=w281, "Method"=w278, "Update"=FALSE) -> (w279:T20)
                  }
                }
              }
              event "Parameter Table": Value Change {
                w291 = TRUE ("Update")
                n214 = event-data() -> ("NewVal"=w310:i32)  [unwired: 1 out]
                n215 = Unbundle By Name(w294) -> ("Method.Lenses"=w307:T5[])
                n216 = Array Size(array=w307) -> (size(s)=w298:i32)
                n217 = Subtract(x=w298, y=7) -> (x-y=w308:i32)
                n218 = In Range and Coerce(upper limit=w308, x=w310, lower limit=0) -> (coerced(x)=w295:i32)  [unwired: 1 out]
                n219 = local write "Parameter Table"(w295) -> ()
                n220 = property on="Parameter Table" class="MCListbox (strict)"() -> ("Item Names"=w299:string[][])  [unwired: 2 in, 2 out]
                n221 = Index Array(array=w299, index (row)=w295, index (col)=0 ("disabled index (col)")) -> (element=w301:string)
                n222 = call "_Get Lens Configuration.vi"("Name"=w301) -> ("Config Row#"=w292:i32, "Lens Configuration"=w296:T19)  [unwired: 1 in, 4 out]
                n223 = Index Array(array=w307, index=w292) -> (element=w306:T5)
                n224 = Unbundle By Name(w296) -> ("Ch#"=w305:u8, "Slope"=w304:dbl, "Offset"=w303:dbl)
                n225 = Unbundle By Name(w306) -> ("Value 1"=w302:dbl)
                n226 = case shown="2, 5" w305 {
                  tunnel: w302 -> [w315 w318 w321]
                  tunnel: [w312 w317 w320] -> w311
                  tunnel: w304 -> [w314 _ _]
                  tunnel: w303 -> [w313 _ _]
                  frame Default {
                    n227 = Multiply(x=w315, y=w314) -> (x*y=w316:dbl)
                    n228 = Add(x=w316, y=w313) -> (x+y=w312:dbl)
                  }
                  frame 1, 4 {
                    n229 = global read "_Global Configuration.vi" "Calibration"() -> (w319:dbl[][])
                    n230 = call "_Convert Mass to DAC.vi"("Calibration Table"=w319, "Mass"=w318) -> ("DAC Value"=w317:dbl)  [unwired: 2 in, 3 out]
                  }
                  frame 2, 5 {
                    n231 = global read "_Global Configuration.vi" "Calibration 2"() -> (w322:dbl[][])
                    n232 = call "_Convert Mass to DAC.vi"("Calibration Table"=w322, "Mass"=w321) -> ("DAC Value"=w320:dbl)  [unwired: 2 in, 3 out]
                  }
                }
                n233 = Bundle By Name(cluster=w294, "Update"=w291, "BlockUpdate"=w291) -> (w293:T20)
                n234 = local write "DAC Value"(w311) -> ()
                n235 = local write "Count1"(w302) -> ()
              }
              event "Run 2": Value Change {
                n236 = event-data() -> ()  [unwired: 7 out]
                n237 = stacked-sequence {
                  tunnel: w328 -> [_ _ w352 _ _]
                  tunnel: w327 -> [w334 _ _ _ _]
                  tunnel: w326 -> [_ w339 _ _ _]
                  tunnel: [_ w338 _ _ _] -> w324
                  frame #0 {
                    w330 = T24 1 items=["Diagnostics", "Tune", "Acquisition"] ("RunModule")
                    w329 = u8 1 ("Disabled")
                    n238 = call <vilib>:"Set Busy.vi"() -> ()  [unwired: 4 in, 8 out]
                    n239 = global write "_Global Configuration.vi" "ScanParam"("Scan Parameter with Mass") -> ()
                    n240 = property on="Run 2" class="Bool"("Visible"=FALSE) -> ()  [unwired: 2 in, 2 out]
                    n241 = property on="Cancel" class="Bool"("Visible"=TRUE) -> ()  [unwired: 2 in, 2 out]
                    n242 = global write "_Global Configuration.vi" "RunModule"(w330) -> ()
                    n243 = call "_Remote BlockUpdate.vi"() -> ()  [unwired: 3 in, 5 out]
                    n244 = Flush Queue(queue=w334) -> ()  [unwired: 1 in, 3 out]
                    n245 = property on="Scan#" class="DigNum (strict)"("Disabled"=w329) -> ()  [unwired: 2 in, 2 out]
                    n246 = property on="Acquire" class="Bool (strict)"("Disabled"=w329) -> ()  [unwired: 2 in, 2 out]
                    n247 = property on="MCA" class="Bool (strict)"("Disabled"=w329) -> ()  [unwired: 2 in, 2 out]
                    n248 = property on="Scan Parameter with Mass" class="Bool (strict)"("Disabled"=w329) -> ()  [unwired: 2 in, 2 out]
                    n249 = property on="Scan Type" class="Enum (strict)"("Disabled"=w329) -> ()  [unwired: 2 in, 2 out]
                    n250 = property on="Delay Time (ms)" class="DigNum (strict)"("Disabled"=w329) -> ()  [unwired: 2 in, 2 out]
                    n251 = property on="Polarity" class="RadioBtnsControl (strict)"("Disabled"=w329) -> ()  [unwired: 2 in, 2 out]
                    n252 = property on="CEM POL" class="Bool (strict)"("Disabled"=w329) -> ()  [unwired: 2 in, 2 out]
                    n253 = property on="Q1DC POL" class="Bool (strict)"("Disabled"=w329) -> ()  [unwired: 2 in, 2 out]
                    n254 = property on="Q2DC POL" class="Bool (strict)"("Disabled"=w329) -> ()  [unwired: 2 in, 2 out]
                    n255 = property on="Run Duration (s)" class="DigNum (strict)"("Disabled"=w329) -> ()  [unwired: 2 in, 2 out]
                    n256 = property on="Ramping Parameter" class="Ring (strict)"("Disabled"=w329) -> ()  [unwired: 2 in, 2 out]
                    n257 = property on="Perform Parameter Ramp" class="Bool (strict)"("Disabled"=w329) -> ()  [unwired: 2 in, 2 out]
                    n258 = property on="Start Mass (amu)" class="DigNum (strict)"("Disabled"=w329) -> ()  [unwired: 2 in, 2 out]
                    n259 = property on="Step Mass (amu)" class="DigNum (strict)"("Disabled"=w329) -> ()  [unwired: 2 in, 2 out]
                    n260 = property on="Stop Mass (amu)" class="DigNum (strict)"("Disabled"=w329) -> ()  [unwired: 2 in, 2 out]
                    n261 = property on="Dwell Time (ms)" class="DigNum (strict)"("Disabled"=w329) -> ()  [unwired: 2 in, 2 out]
                    n262 = property on="Resolution (Q1/Q2)" class="Ring (strict)"("Disabled"=w329) -> ()  [unwired: 2 in, 2 out]
                    n263 = property on="Pause Time (ms)" class="DigNum (strict)"("Disabled"=w329) -> ()  [unwired: 2 in, 2 out]
                    n264 = property on="# of Cycles" class="DigNum (strict)"("Disabled"=w329) -> ()  [unwired: 2 in, 2 out]
                    n265 = property on="Fixed Mass (amu)" class="DigNum (strict)"("Disabled"=w329) -> ()  [unwired: 2 in, 2 out]
                    n266 = property on="Insert Row" class="Bool"("Disabled"=w329) -> ()  [unwired: 2 in, 2 out]
                    n267 = property on="Delete Row" class="Bool"("Disabled"=w329) -> ()  [unwired: 2 in, 2 out]
                    n268 = property on="MR Parameters" class="Bool"("Disabled"=w329) -> ()  [unwired: 2 in, 2 out]
                    n269 = property on="Stop Value" class="DigNum (strict)"("Disabled"=w329) -> ()  [unwired: 2 in, 2 out]
                    n270 = property on="Step Value" class="DigNum (strict)"("Disabled"=w329) -> ()  [unwired: 2 in, 2 out]
                    n271 = property on="Start Value" class="DigNum (strict)"("Disabled"=w329) -> ()  [unwired: 2 in, 2 out]
                  }
                  frame #1 {
                    n272 = case shown="True" "Acquire" {
                      tunnel: w339 -> [w340 w345]
                      tunnel: [w340 w342] -> w338
                      frame False {
                      }
                      frame True {
                        n273 = local read "Data File:"() -> (w346:path)
                        n274 = call "_Get File.vi"("Start Path"=w346) -> ("Seleted File"=w347:path, "Succeeded"=w343:bool)  [unwired: 5 in, 2 out]
                        n275 = local write "Acquire"(w343) -> ()
                        n276 = case shown="True" w343 {
                          tunnel: w347 -> [_ w349]
                          tunnel: w346 -> [w348 _]
                          tunnel: [w348 w349] -> w344
                          frame False {
                          }
                          frame True {
                            n277 = local write "Data File:"(w349) -> ()
                          }
                        }
                        n278 = Bundle By Name(cluster=w345, "Method.Data Path"=w344, "Method.Acquire"=w343) -> (w342:T20)
                        n279 = Unbundle By Name(w342) -> ("Method"=w341:T4)
                        n280 = local write "Method"(w341) -> ()
                      }
                    }
                    n281 = call "_Launch Dynamic VI.vi"("VI Name"=path "Real Time Display.vi" ("name or relative path")) -> ()  [unwired: 3 in, 1 out]
                    n282 = global write "_Global Configuration.vi" "Run"(TRUE ("Update")) -> ()
                  }
                  frame #2 {
                    w351 = FALSE ("Wait until done")
                    n283 = invoke class="VI" method="Run VI"(reference=w352, "Wait until done"=w351, "Auto Dispose Ref"=w351) -> ()  [unwired: 2 in, 5 out]
                    n284 = local write "Scan#"(u32 0 ("Scan#")) -> ()
                  }
                  frame #3 {
                    n285 = Wait (ms)(milliseconds to wait=u32 800) -> ()  [unwired: 1 out]
                  }
                  frame #4 {
                    n286 = call <vilib>:"Unset Busy.vi"() -> ()  [unwired: 2 in, 10 out]
                  }
                }
                n287 = Bundle By Name(cluster=w324, "Running"=TRUE) -> (w323:T20)
              }
              event "Cancel": Value Change {
                n288 = event-data() -> ()  [unwired: 7 out]
                n289 = stacked-sequence {
                  tunnel: w356 -> [_ w359 _]
                  tunnel: [_ w359 _] -> w355
                  tunnel: w354 -> [_ w358 _]
                  frame #0 {
                    n290 = call <vilib>:"Set Busy.vi"() -> ()  [unwired: 4 in, 8 out]
                    n291 = global write "_Global Configuration.vi" "Run"(FALSE ("Update")) -> ()
                  }
                  frame #1 {
                    n292 = while {
                      tunnel: w358 -> [w364]
                      stop <- w361 stop-if-true
                      n293 = property class="VI"(reference=w364) -> ("Exec.State"=w363:T14)  [unwired: 1 in, 2 out]
                      n294 = Wait (ms)(milliseconds to wait=u32 180) -> ()  [unwired: 1 out]
                      n295 = Equal?(x=w363, y=T14."Idle") -> (x = y?=w361:bool)
                    }
                  }
                  frame #2 {
                    n296 = call "_Remote Wait Until Done.vi"() -> ("error out"=w365:errorcluster)  [unwired: 2 in, 1 out]
                    n297 = call "_Remote Park Lens.vi"("error in"=w365) -> ()  [unwired: 1 in, 6 out]
                    n298 = call <vilib>:"Unset Busy.vi"() -> ()  [unwired: 2 in, 10 out]
                  }
                }
              }
              event "BloUpdate": Value Change {
                w369 = FALSE
                n299 = event-data() -> ()  [unwired: 7 out]
                n300 = Unbundle By Name(w368) -> ("Running"=w370:bool, "BlockUpdate"=w366:bool)
                n301 = stacked-sequence {
                  seq-local: [_ w373 _ _] -> [_ _ _ w383]
                  tunnel: w370 -> [_ w372 _ _]
                  tunnel: w366 -> [_ w371 _ _]
                  frame #0 {
                    n302 = call <vilib>:"Set Busy.vi"() -> ()  [unwired: 4 in, 8 out]
                  }
                  frame #1 {
                    n303 = case shown="True" w371 {
                      tunnel: [w375 w382] -> w373
                      tunnel: w372 -> [w374 w381]
                      frame False {
                        n304 = local read "Parameter Table"() -> (w380:i32)
                        n305 = local read "DAC Value"() -> (w376:i32)
                        n306 = property on="Parameter Table" class="MCListbox (strict)"() -> ("Item Names"=w378:string[][])  [unwired: 2 in, 2 out]
                        n307 = Index Array(array=w378, index (row)=w380, index (col)=0 ("disabled index (col)")) -> (element=w377:string)
                        n308 = call "_Remote Single Update.vi"("DACValue"=w376, "ParamName"=w377, "Running"=w374) -> ("error out"=w375:errorcluster)  [unwired: 1 in, 3 out]
                      }
                      frame True {
                        n309 = call "_Remote BlockUpdate.vi"("Running"=w381) -> ("error out"=w382:errorcluster)  [unwired: 2 in, 4 out]
                      }
                    }
                  }
                  frame #2 {
                    n310 = call <vilib>:"Unset Busy.vi"() -> ()  [unwired: 2 in, 10 out]
                  }
                  frame #3 {
                    n311 = call "_Handle Error.vi"("error in (no error)"=w383) -> ()  [unwired: 2 in, 5 out]
                  }
                }
                n312 = local write "BloUpdate"(w369) -> ()
                n313 = Bundle By Name(cluster=w368, "BlockUpdate"=w369) -> (w367:T20)
              }
              event "NewMethod": Value Change {
                w391 = 0 ("Value (Signaling)")
                n314 = event-data() -> ()  [unwired: 7 out]
                n315 = local write "NewMethod"(FALSE) -> ()
                n316 = Unbundle By Name(w393) -> ("Running"=w385:bool, "Method"=w395:T4)
                n317 = global read "_Global Configuration.vi" "Configuration 2"() -> (w388:T18)
                n318 = property on="Parameter Table" class="MCListbox (strict)"("Value (Signaling)"=w391) -> ()  [unwired: 2 in, 2 out]
                n319 = property on="Mass Range" class="MCListbox (strict)"("Value"=w391) -> ()  [unwired: 2 in, 2 out]
                n320 = Unbundle By Name(w388) -> ("Table"=w387:T19[])
                n321 = Unbundle By Name(w395) -> ("Negative"=w384:bool, "Run Mode"=w389:T2, "Fixed Mass (amu)"=w390:dbl, "Acquire"=w405:bool, "MCA"=w404:bool, "Q1 POL"=w386:bool, "Q3 POL"=w406:bool, "Averaging"=w400:bool, "Log Scale"=w401:bool, "CPS"=w402:bool, "Data Path"=w403:path, "Lenses"=w396:T5[])  [unwired: 2 out]
                n322 = Array Size(array=w396) -> (size(s)=w398:i32)
                n323 = Array Size(array=w387) -> (size(s)=w399:i32)
                n324 = Not Equal?(x=w398, y=w399) -> (x != y?=w397:bool)
                n325 = case shown="True" w397 {
                  tunnel: w387 -> [_ w413]
                  tunnel: [w408 w411] -> w394
                  tunnel: w396 -> [w408 _]
                  tunnel: w384 -> [_ w410]
                  frame False {
                  }
                  frame True {
                    n326 = for {
                      tunnel: w413 -> [w417] mode=indexing
                      tunnel: T5 {"Scan Type"=0, "Scans"=1, "Time 1"=1.0, "Time 2"=1.0, "Value 1"=0.0, "Value 2"=0.0, "Step Size"=1.0} ("Lenses") -> [w418]
                      tunnel: [w416] -> w411 mode=indexing
                      tunnel: w410 -> [w415]
                      n327 = case shown="False" w415 {
                        tunnel: w417 -> [w420 w422]
                        tunnel: [w419 w421] -> w414
                        frame False {
                          n328 = Unbundle By Name(w420) -> ("Def+"=w419:dbl)
                        }
                        frame True {
                          n329 = Unbundle By Name(w422) -> ("Def-"=w421:dbl)
                        }
                      }
                      n330 = Bundle By Name(cluster=w418, "Value 1"=w414, "Value 2"=w414) -> (w416:T5)
                    }
                    n331 = One Button Dialog(message="Default parameter values applied.") -> ()  [unwired: 2 out]
                  }
                }
                n332 = stacked-sequence {
                  tunnel: w386 -> [w428 _ _]
                  tunnel: w406 -> [w427 _ _]
                  tunnel: w405 -> [_ _ w458]
                  tunnel: w404 -> [_ _ w457]
                  tunnel: w403 -> [_ w451 _]
                  tunnel: w402 -> [_ w450 _]
                  tunnel: w401 -> [_ w449 _]
                  tunnel: w400 -> [_ w448 _]
                  tunnel: w390 -> [_ _ w456]
                  tunnel: w389 -> [_ _ w455]
                  tunnel: w385 -> [w425 _ _]
                  tunnel: w384 -> [_ w447 _]
                  frame #0 {
                    n333 = local write "Q1DC POL"(w428) -> ()
                    n334 = Number To Boolean Array(number=u16 0) -> (Boolean array=w435:bool[])
                    n335 = local read "Scan Type"() -> (w426:T2)
                    n336 = local write "Q2DC POL"(w427) -> ()
                    n337 = case shown="\"Q1 Scan\", \"Q1 SRM\"" w426 {
                      tunnel: [w440 _ TRUE] -> w424
                      tunnel: [w440 TRUE _] -> w423
                      frame Default {
                        w440 = TRUE
                        # "MS/MS"
                      }
                      frame "Q1 Scan", "Q1 SRM" {
                        # "Q1"
                      }
                      frame "Q2 Scan", "Q2 SRM" {
                        # "Q2"
                      }
                    }
                    n338 = Replace Array Subset(array=w435, new element #1=w428, index #1=0 ("index"), new element #2=w427, index #2=1 ("index"), new element #3=w423, index #3=2 ("index"), new element #4=w424, index #4=3 ("index")) -> (w430:bool[])
                    n339 = Boolean Array To Number(Boolean array=w430) -> (number=w429:u16)
                    n340 = case shown="False" w425 {
                      tunnel: [w438 _] -> _
                      tunnel: w429 -> [w437 _]
                      frame False {
                        n341 = call "_Remote Communicate.vi"("DC Param"=w437, "Command"=_RT_Command."Set Pol and DC") -> ("error out"=w438:errorcluster)  [unwired: 4 in, 3 out]
                      }
                      frame True {
                      }
                    }
                  }
                  frame #1 {
                    n342 = local write "Averaging"(w448) -> ()
                    n343 = local write "Log Scale"(w449) -> ()
                    n344 = local write "CPS"(w450) -> ()
                    n345 = call "_Read Spectrum File.vi"("advisory dialog? (display:T)"=FALSE, "start path  (Not A Path)"=w451) -> ("new file path"=→"Data File:":path, "Scan# out"=w452:u32)  [unwired: 1 in, 5 out]
                    n346 = local write "Scan#"(w452) -> ()
                    n347 = Select(t=enum32{"Positive Ions", "Negative Ions"}."Negative Ions", s=w447, f=enum32{"Positive Ions", "Negative Ions"}."Positive Ions" ("Polarity")) -> (s? t:f=w444:enum32{"Positive Ions", "Negative Ions"})
                    n348 = local write "Polarity"(w444) -> ()
                    n349 = property on="Use Pol Swap Options from Config" class="Bool (strict)"("Value (Signaling)"=FALSE) -> ()  [unwired: 2 in, 2 out]
                  }
                  frame #2 {
                    n350 = local write "Acquire"(w458) -> ()
                    n351 = local write "MCA"(w457) -> ()
                    n352 = local write "Fixed Mass (amu)"(w456) -> ()
                    n353 = global read "_Global Configuration.vi" "Spectrum"() -> (w459:i32[])
                    n354 = property on="Scan Type" class="Enum (strict)"("Val(Sgnl)"=w455) -> ()  [unwired: 2 in, 2 out]
                    n355 = call "_Update Display Property 2.vi"("Spectrum in"=w459) -> ()  [unwired: 7 out]
                  }
                }
                n356 = Bundle By Name(cluster=w393, "Method.Lenses"=w394) -> (w392:T20)
              }
              event "Count1": Value Change {
                # "perform single update only"
                n357 = event-data() -> ()  [unwired: 2 out]
                n358 = Bundle By Name(cluster=w462, "Update"=TRUE) -> (w461:T20)
              }
              event "Use Pol Swap Options from Config": Value Change {
                n359 = event-data() -> ("NewVal"=w478:bool)  [unwired: 1 out]
                n360 = global read "_Global Configuration.vi" "Configuration 2"() -> (w463:T18)
                n361 = Unbundle By Name(w463) -> ("Instrument"=w464:string[])
                n362 = local read "Polarity"() -> (w472:enum32{"Positive Ions", "Negative Ions"})
                n363 = Equal?(x=w472, y=enum32{"Positive Ions", "Negative Ions"}."Positive Ions" ("Polarity")) -> (x = y?=w466:bool)
                n364 = Index Array(array=w464, index=13) -> (element=w475:string)
                n365 = Decimal String To Number(string=w475) -> (number=w476:i32)  [unwired: 3 out]
                n366 = Number To Boolean Array(number=w476) -> (Boolean array=w473:bool[])
                n367 = Select(t=0, s=w466, f=2) -> (s? t:f=w465:i32)
                n368 = case shown="False" w478 {
                  tunnel: w477 -> [w496 _]
                  tunnel: w473 -> [w494 w504]
                  tunnel: [w489 w503] -> w470
                  tunnel: [w488 w502] -> w469
                  tunnel: w465 -> [w493 w501]
                  tunnel: w464 -> [w480 _]
                  tunnel: w463 -> [w485 _]
                  frame False {
                    n369 = Unbundle By Name(w496) -> ("Method"=w495:T4)
                    n370 = Initialize Array("", 16 ("dimension size")) -> (w481:string[])
                    n371 = Unbundle By Name(w495) -> ("Q1 POL"=w489:bool, "Q3 POL"=w488:bool)
                    n372 = Replace Array Subset(array=w481, new element=w480) -> (w479:string[])  [unwired: 1 in]
                    n373 = local write "Q1DC POL"(w489) -> ()
                    n374 = local write "Q2DC POL"(w488) -> ()
                    n375 = Replace Array Subset(array=w494, new element #1=w489, index #1=w493, new element #2=w488) -> (w492:bool[])  [unwired: 1 in]
                    n376 = Boolean Array To Number(Boolean array=w492) -> (number=w491:u32)
                    n377 = To Long Integer(number=w491) -> (32bit integer=w490:i32)
                    n378 = Number To Decimal String(number=w490) -> (decimal integer string=w486:string)  [unwired: 1 out]
                    n379 = Replace Array Subset(array=w479, new element=w486, index=13) -> (w484:string[])
                    n380 = stacked-sequence {
                      tunnel: w485 -> [w499 _]
                      tunnel: w484 -> [w498 _]
                      frame #0 {
                        n381 = Bundle By Name(cluster=w499, "Instrument"=w498) -> (w497:T18)
                        n382 = global write "_Global Configuration.vi" "Configuration 2"(w497) -> ()
                      }
                      frame #1 {
                        n383 = call "_Remote Communicate.vi"("Command"=_RT_Command."Update Config") -> ()  [unwired: 5 in, 4 out]
                      }
                    }
                  }
                  frame True {
                    n384 = Index Array(array=w504, index #1=w501) -> (element #1=w503:bool, element #2=w502:bool)  [unwired: 1 in]
                  }
                }
                n385 = local write "Q1DC POL"(w470) -> ()
                n386 = local write "Q2DC POL"(w469) -> ()
              }
              event "Swtich Polarity": Value Change {
                n387 = event-data() -> ()  [unwired: 7 out]
                n388 = Unbundle By Name(w507) -> ("Method.Lenses"=w505:T5[], "Running"=w506:bool)
                n389 = case shown="False" w506 {
                  tunnel: w507 -> [w519 w522]
                  tunnel: [w517 w522] -> w508
                  tunnel: w505 -> [w516 _]
                  frame False {
                    w509 = TRUE
                    n390 = local read "Parameter Table"() -> (w510:i32)
                    n391 = property on="Parameter Table" class="MCListbox (strict)"() -> ("Item Names"=w512:string[][])  [unwired: 2 in, 2 out]
                    n392 = Index Array(array=w512, index (row)=w510, index (col)=0 ("disabled index (col)")) -> (element=w514:string)
                    n393 = call "_Get Lens Configuration.vi"("Name"=w514) -> ("Lens Configuration"=w511:T19)  [unwired: 1 in, 5 out]
                    n394 = Unbundle By Name(w511) -> ("Ch#"=w515:u8)
                    n395 = call "_Switch Polarity.vi"("Lenses"=w516) -> ("Lenses 2"=w518:T5[])  [unwired: 5 in, 2 out]
                    n396 = case shown="Default" w515 {
                      frame Default {
                        n397 = local read "Count1"() -> (w521:dbl)
                        n398 = Negate(x=w521) -> (-x=w520:dbl)
                        n399 = local write "Count1"(w520) -> ()
                      }
                      frame 1..5, 7, 9, 26..94 {
                      }
                    }
                    n400 = Bundle By Name(cluster=w519, "Method.Lenses"=w518, "Update"=w509, "BlockUpdate"=w509) -> (w517:T20)
                  }
                  frame True {
                    n401 = One Button Dialog(message="You must wait until the run is finish before you can switch lens polarity.") -> ()  [unwired: 2 out]
                  }
                }
              }
              event "Q1DC POL", "Q2DC POL": Value Change {
                w540 = TRUE
                n402 = event-data() -> ()  [unwired: 2 out]
                n403 = local read "Scan Type"() -> (w528:T2)
                n404 = Unbundle By Name(w541) -> ("Running"=w529:bool)
                n405 = case shown="\"Q2 Scan\", \"Q2 SRM\"" w528 {
                  tunnel: [w544 _ TRUE] -> w526
                  tunnel: [w544 TRUE _] -> w527
                  frame Default {
                    w544 = TRUE
                    # "MS/MS"
                  }
                  frame "Q1 Scan", "Q1 SRM" {
                    # "Q1"
                  }
                  frame "Q2 Scan", "Q2 SRM" {
                    # "Q2"
                  }
                }
                n406 = Number To Boolean Array(number=u16 0) -> (Boolean array=w538:bool[])
                n407 = Replace Array Subset(array=w538, new element #1="Q1DC POL", index #1=0 ("index"), new element #2="Q2DC POL", index #2=1 ("index"), new element #3=w527, index #3=2 ("index"), new element #4=w526, index #4=3 ("index")) -> (w533:bool[])
                n408 = Boolean Array To Number(Boolean array=w533) -> (number=w532:u16)
                n409 = case shown="False" w529 {
                  tunnel: [w547 _] -> w525
                  tunnel: w532 -> [w548 _]
                  frame False {
                    n410 = call "_Remote Communicate.vi"("DC Param"=w548, "Command"=_RT_Command."Set Pol and DC") -> ("error out"=w547:errorcluster)  [unwired: 4 in, 3 out]
                  }
                  frame True {
                  }
                }
                n411 = Bundle By Name(cluster=w541, "Method.Q1 POL"="Q1DC POL", "Method.Q3 POL"="Q2DC POL", "Method.Q1 RF  EN"=w540, "Method.Q3 RF  EN"=w540) -> (w542:T20)
                n412 = property on="Use Pol Swap Options from Config" class="Bool (strict)"("Value (Signaling)"=FALSE) -> ()  [unwired: 2 in, 2 out]
                n413 = Unbundle By Name(w542) -> ("Method"=w543:T4)
                n414 = call "_Handle Error.vi"("error in (no error)"=w525) -> ()  [unwired: 2 in, 5 out]
                n415 = local write "Method"(w543) -> ()
              }
              event "Export Settings": Value Change {
                n416 = event-data() -> ()  [unwired: 2 out]
                n417 = global read "_Global Configuration.vi" "Method Refnum"() -> (w560:refnum<vi>)
                n418 = property class="Clust (strict)"(reference=w560) -> ("Value"=w562:T25)  [unwired: 1 in, 2 out]
                n419 = global read "_Global Configuration.vi" "Configuration 2"() -> (w561:T18)
                n420 = Unbundle By Name(w561) -> ("Table"=w559:T19[])
                n421 = Unbundle By Name(w562) -> ("Lenses"=w558:T5[])
                n422 = for {
                  tunnel: w559 -> [w574] mode=indexing
                  tunnel: w558 -> [w573] mode=indexing
                  tunnel: [w566] -> w557 mode=indexing
                  # "For Each Channel"
                  n423 = Unbundle By Name(w573) -> ("Value 1"=w572:dbl)
                  n424 = Unbundle By Name(w574) -> ("Ch#"=w570:u8, "Name"=w568:string)
                  n425 = Number To Fractional String(number=w572, precision (6)=i16 2) -> (F-format string=w567:string)  [unwired: 2 out]
                  n426 = Number To Decimal String(number=w570) -> (decimal integer string=w569:string)  [unwired: 1 out]
                  n427 = Build Array(w569, w568, w567) -> (w566:string[])
                }
                n428 = call "_Get File.vi"("For Write (T)"=TRUE, "select mode (new or existing)"=T15."new or existing file", "default name"="My Tune Settings", "extension (isd)"="*.txt" ("pattern (all files)"), "prompt"="Please enter an export file name.") -> ("Seleted File"=w550:path, "Succeeded"=w551:bool)  [unwired: 1 in, 2 out]
                n429 = case shown="True" w551 {
                  tunnel: w557 -> [_ w565]
                  tunnel: w550 -> [_ w564]
                  frame False {
                  }
                  frame True {
                    n430 = call "_Export Table To Text File.vi"("2D data"=w565, "file path (dialog if empty)"=w564) -> ()  [unwired: 4 in, 3 out]
                  }
                }
              }
              event "CPS", "Averaging", "Log Scale": Value Change {
                n431 = event-data() -> ()  [unwired: 7 out]
                n432 = stacked-sequence {
                  tunnel: w576 -> [w582 w584]
                  tunnel: [w578 _] -> w575
                  frame #0 {
                    n433 = Bundle By Name(cluster=w582, "Method.Averaging"="Averaging", "Method.Log Scale"="Log Scale", "Method.CPS"="CPS") -> (w578:T20)
                    n434 = Unbundle By Name(w578) -> ("Method"=w577:T4)
                    n435 = local write "Method"(w577) -> ()
                  }
                  frame #1 {
                    n436 = Unbundle By Name(w584) -> ("Running"=w583:bool)
                    n437 = case shown="False" w583 {
                      frame False {
                        n438 = global read "_Global Configuration.vi" "Spectrum"() -> (w585:i32[])
                        n439 = call "_Update Display Property 2.vi"("Spectrum in"=w585) -> ()  [unwired: 7 out]
                      }
                      frame True {
                      }
                    }
                  }
                }
              }
              event "Acquire", "MCA", "Fixed Mass (amu)": Value Change {
                n440 = event-data() -> ()  [unwired: 7 out]
                n441 = local read "Acquire"() -> (w590:bool)
                n442 = Bundle By Name(cluster=w591, "Method.Acquire"=w590, "Method.MCA"="MCA", "Method.Fixed Mass (amu)"="Fixed Mass (amu)") -> (w587:T20)
                n443 = Unbundle By Name(w587) -> ("Method"=w588:T4)
                n444 = local write "Method"(w588) -> ()
              }
              event "Polarity": Value Change {
                w594 = TRUE  # Running?
                n445 = event-data() -> ()  [unwired: 7 out]
                n446 = Equal?(x="Polarity", y=enum32{"Positive Ions", "Negative Ions"}."Negative Ions") -> (x = y?=w595:bool)
                n447 = case shown="False" w594 {
                  tunnel: w595 -> [w600 _]
                  frame False {
                    n448 = stacked-sequence {
                      tunnel: w600 -> [_ _ _ w613]
                      frame #0 {
                        n449 = call <vilib>:"Set Busy.vi"() -> ()  [unwired: 4 in, 8 out]
                      }
                      frame #1 {
                        w608 = u16 0 ("Set Value")
                        n450 = call "_Remote Set PIC.vi"("Set Value"=w608, "PIC Channel"=_PIC_Channel."Corona +HV") -> ("error out"=w605:errorcluster)  [unwired: 1 in, 4 out]
                        n451 = call "_Remote Set PIC.vi"("error in (no error)"=w605, "Set Value"=w608, "PIC Channel"=_PIC_Channel."Corona +HV") -> ("error out"=w604:errorcluster)  [unwired: 4 out]
                        n452 = call "_Remote Set PIC.vi"("error in (no error)"=w604, "Set Value"=w608, "PIC Channel"=_PIC_Channel."Corona +HV") -> ("error out"=w603:errorcluster)  [unwired: 4 out]
                        n453 = call "_Remote Set PIC.vi"("error in (no error)"=w603, "Set Value"=w608, "PIC Channel"=_PIC_Channel."Corona +HV") -> ("error out"=w609:errorcluster)  [unwired: 4 out]
                        n454 = call "_Remote Set CEM.vi"("error in"=w609) -> ()  [unwired: 2 in, 5 out]
                      }
                      frame #2 {
                        n455 = Wait (ms)(milliseconds to wait=u32 1000) -> ()  [unwired: 1 out]
                      }
                      frame #3 {
                        n456 = Not(x=w613) -> (.not. x?=w612:bool)
                        n457 = Boolean To (0,1)(Boolean=w612) -> (0, 1=w611:i16)
                        n458 = call "_Remote Communicate.vi"("DC Param"=w611, "Command"=_RT_Command."Set All Pol") -> ()  [unwired: 4 in, 4 out]
                        n459 = call <vilib>:"Unset Busy.vi"() -> ()  [unwired: 2 in, 10 out]
                      }
                    }
                  }
                  frame True {
                  }
                }
                n460 = Bundle By Name(cluster=w596, "Method.Negative"=w595) -> (w598:T20)
                n461 = property on="Use Pol Swap Options from Config" class="Bool (strict)"("Value (Signaling)"=FALSE) -> ()  [unwired: 2 in, 2 out]
                n462 = Unbundle By Name(w598) -> ("Method"=w599:T4)
                n463 = local write "Method"(w599) -> ()
              }
              event "Center/Width": Value Change {
                n464 = local read "Center/Width"() -> (w618:bool)
                n465 = event-data() -> ()  [unwired: 2 out]
                n466 = local read "Scan Type"() -> (w619:T2)
                n467 = case shown="\"Product Scan\", Default" w619 {
                  selector: w619 -> [_ w645 _ _ _]
                  tunnel: [_ w643 _ _ _] -> w626
                  tunnel: [w629 w649 string[] ["\n#", "Q1\n(amu)", "Q2\n(amu)", "Dwell\n(ms)", "", "", "Res"] ("Column Header Strings[]") string[] ["\n#", "Q1\n(amu)", "Ignored", "Dwell\n(ms)", "", "", "Res"] ("Column Header Strings[]") string[] ["\n#", "Ignored", "Q2\n(amu)", "Dwell\n(ms)", "", "", "Res"] ("Column Header Strings[]")] -> w625
                  tunnel: ["Step Mass (amu)" "Step Mass (amu)" "Not Used" "Not Used" "Not Used"] -> w624
                  tunnel: [w630 w647 "Q2 Mass (amu)" "Not Used" "Q2 Mass (amu)"] -> w623
                  tunnel: [w631 w646 "Q1 Mass (amu)" "Q1 Mass (amu)" "Not Used"] -> w622
                  tunnel: ["Fixed Mass (amu)" w644 "Fixed Mass (amu)" "Fixed Mass (amu)" "Fixed Mass (amu)"] -> w621
                  tunnel: w618 -> [w632 w642 _ _ _]
                  tunnel: [w633 w643 w659 _ TRUE] -> w617
                  tunnel: [w633 w643 w659 TRUE _] -> w616
                  tunnel: [w633 w643 _ _ _] -> w615
                  frame "Q1 Scan", "Q2 Scan" {
                    w633 = TRUE
                    n468 = case shown="False" w632 {
                      tunnel: [string[] ["\n#", "Center\n(amu)", "Width\n(amu)", "Step\n(amu)", "Dwell\n(ms)", "# of\nSteps", "Res"] ("Column Header Strings[]") string[] ["\n#", "Start\n(amu)", "Stop\n(amu)", "Step\n(amu)", "Dwell\n(ms)", "# of\nSteps", "Res"] ("Column Header Strings[]")] -> w629
                      tunnel: ["Width (amu)" "Stop Mass (amu)"] -> w630
                      tunnel: ["Center Mass (amu)" "Start Mass (amu)"] -> w631
                      frame True {
                      }
                      frame False {
                      }
                    }
                  }
                  frame "Product Scan", Default {
                    w643 = TRUE
                    n469 = case shown="True" w642 {
                      tunnel: [string[] ["\n#", "Center\n(amu)", "Width\n(amu)", "Step\n(amu)", "Dwell\n(ms)", "# of\nSteps", "Res"] ("Column Header Strings[]") string[] ["\n#", "Start\n(amu)", "Stop\n(amu)", "Step\n(amu)", "Dwell\n(ms)", "# of\nSteps", "Res"] ("Column Header Strings[]")] -> w649
                      tunnel: ["Width (amu)" "Stop Mass (amu)"] -> w647
                      tunnel: ["Center Mass (amu)" "Start Mass (amu)"] -> w646
                      frame True {
                      }
                      frame False {
                      }
                    }
                    n470 = case shown="\"Precursor Scan\"" w645 {
                      tunnel: ["Precursor Mass (amu)" "Neutral Mass (amu)" "Daughter Mass (amu)"] -> w644
                      frame "Product Scan" {
                      }
                      frame Default {
                      }
                      frame "Precursor Scan" {
                      }
                    }
                  }
                  frame "MRM (Q1/Q2)" {
                    w659 = TRUE
                  }
                  frame "Q1 SRM" {
                  }
                  frame "Q2 SRM" {
                  }
                }
                n471 = Bundle By Name(cluster=w628, "Method.Run Mode"=w619) -> (w627:T20)
                n472 = local read "Mass Range"() -> (w620:i32)
                n473 = property on="Fixed Mass (amu)" class="DigNum (strict)"("Visible"=w626, "Caption.Text"=w621) -> ()  [unwired: 2 in, 2 out]
                n474 = property on="Mass Range" class="MCListbox (strict)"("ColHdrString"=w625, "Val(Sgnl)"=w620) -> ()  [unwired: 2 in, 2 out]
                n475 = property on="Start Mass (amu)" class="DigNum (strict)"("Caption.Text"=w622, "Visible"=w616) -> ()  [unwired: 2 in, 2 out]
                n476 = property on="Stop Mass (amu)" class="DigNum (strict)"("Caption.Text"=w623, "Visible"=w617) -> ()  [unwired: 2 in, 2 out]
                n477 = property on="Step Mass (amu)" class="DigNum (strict)"("Caption.Text"=w624, "Visible"=w615) -> ()  [unwired: 2 in, 2 out]
                n478 = property on="Center/Width" class="Bool (strict)"("Visible"=w615) -> ()  [unwired: 2 in, 2 out]
              }
              event "Scan#": Value Change {
                n479 = event-data() -> ("NewVal"=w681:u32)  [unwired: 1 out]
                n480 = Unbundle By Name(w678) -> ("Running"=w677:bool)
                n481 = global read "_Global Configuration.vi" "# of Scans"() -> (w680:i32)
                n482 = In Range and Coerce(upper limit=w680, x=w681, lower limit=u32 1) -> (coerced(x)=w679:u32)  [unwired: 1 out]
                n483 = case shown="False" w677 {
                  tunnel: w679 -> [w685 _]
                  frame False {
                    n484 = local read "Data File:"() -> (w687:path)
                    n485 = call "_Read Spectrum File.vi"("advisory dialog? (display:T)"=FALSE, "Scan#"=w685, "start path  (Not A Path)"=w687) -> ("error"=w689:bool, "TIC"=w688:u32, "error out"=w683:errorcluster, "Scan# out"=w686:u32)  [unwired: 3 out]
                    n486 = case shown="False" w689 {
                      tunnel: w688 -> [_ _]
                      tunnel: w686 -> [w691 _]
                      tunnel: w683 -> [_ w692]
                      frame False {
                        n487 = global read "_Global Configuration.vi" "Spectrum"() -> (w690:i32[])
                        n488 = local write "Scan#"(w691) -> ()
                        n489 = call "_Update Display Property 2.vi"("Spectrum in"=w690) -> ()  [unwired: 7 out]
                      }
                      frame True {
                        n490 = call "_Handle Error.vi"("error in (no error)"=w692) -> ()  [unwired: 2 in, 5 out]
                      }
                    }
                  }
                  frame True {
                    n491 = One Button Dialog(message="You must wait until the run is finish before you can load another spectrum.") -> ()  [unwired: 2 out]
                  }
                }
              }
              event "Tab": Value Change {
                n492 = event-data() -> ("NewVal"=w696:T1)  [unwired: 1 out]
                n493 = Equal?(x=w696, y=enum32{"Parameters", "Mass Ranges"}."Mass Ranges") -> (x = y?=w694:bool)
                n494 = case shown="True" w694 {
                  frame False {
                  }
                  frame True {
                    n495 = property on="Mass Range" class="MCListbox (strict)"("Value (Signaling)"="Mass Range") -> ()  [unwired: 2 in, 2 out]
                  }
                }
              }
              event "Mass Range": Value Change {
                n496 = event-data() -> ("NewVal"=w714:i32)  [unwired: 1 out]
                n497 = Unbundle By Name(w727) -> ("Method.Lenses"=w730:T5[], "Method.Mass Ranges"=w715:T6[])
                n498 = call "_Validate Mass Range.vi"("Run Mode"="Scan Type", "Ranges #"=w714, "Mass Ranges"=w715, "Center/Width"="Center/Width") -> ("Cycle Time (ms)"=w700:dbl, "Current Mass Range"=w713:T6, "Mass Ranges Out"=w704:T6[], "Table out"=w710:string[][], "Ramp Time (ms)"=→"Ramp Time (ms)":dbl, "Ranges # Out"=w711:i32)
                n499 = Index Array(array=w730, index=0) -> (element=w728:T5)
                n500 = Unbundle By Name(w728) -> ("Time 1"=w705:dbl, "Time 2"=w702:dbl, "Scans"=w721:i32)
                n501 = property on="Mass Range" class="MCListbox (strict)"("Value"=w711, "Item Names"=w710) -> ()  [unwired: 2 in, 2 out]
                n502 = local write "Delay Time (ms)"(w705) -> ()
                n503 = local write "Pause Time (ms)"(w702) -> ()
                n504 = local write "# of Cycles"(w721) -> ()
                n505 = Bundle By Name(cluster=w727, "Method.Mass Ranges"=w704) -> (w726:T20)
                n506 = Array Size(array=w704) -> (size(s)=w703:i32)
                n507 = Unbundle By Name(w713) -> ("Start"=w723:dbl, "Stop"=w724:dbl, "Step Size"=w716:dbl, "Dwell"=w722:dbl, "Steps"=→"# of Steps":i32, "Res"=w708:T3)
                n508 = Multiply(x=w702, y=w703) -> (x*y=w701:dbl)
                n509 = Add(x=w700, y=w701) -> (x+y=w699:dbl)
                "Cycle Time (ms)" <- w699
                n510 = local write "Resolution (Q1/Q2)"(w708) -> ()
                n511 = local write "Dwell Time (ms)"(w722) -> ()
                n512 = local write "Stop Mass (amu)"(w724) -> ()
                n513 = local write "Step Mass (amu)"(w716) -> ()
                n514 = local write "Start Mass (amu)"(w723) -> ()
                n515 = Unbundle By Name(w726) -> ("Method"=w725:T4)
                n516 = Add(x=w705, y=w699) -> (x+y=w718:dbl)
                n517 = local write "Method"(w725) -> ()
                n518 = Multiply(x=w721, y=w718) -> (x*y=w717:dbl)
                n519 = Divide(x=w717, y=1000.0) -> (x/y=w719:dbl)
                n520 = local write "Run Duration (s)"(w719) -> ()
              }
              event "Run Duration (s)": Value Change {
                n521 = event-data() -> ()  [unwired: 2 out]
                n522 = local read "Delay Time (ms)"() -> (w733:dbl)
                n523 = local read "Cycle Time (ms)"() -> (w734:dbl)
                n524 = Multiply(x="Run Duration (s)", y=1000.0) -> (x*y=w736:dbl)
                n525 = Add(x=w734, y=w733) -> (x+y=w732:dbl)
                n526 = Divide(x=w736, y=w732) -> (x/y=w735:dbl)
                n527 = property on="# of Cycles" class="DigNum (strict)"("Val(Sgnl)"=w735) -> ()  [unwired: 2 in, 2 out]
              }
              event "# of Cycles", "Pause Time (ms)", "Delay Time (ms)": Value Change {
                w749 = 0 ("index")
                w740 = 30000.0 ("upper limit")
                w741 = 0.0 ("lower limit")
                n528 = event-data() -> ()  [unwired: 2 out]
                n529 = Unbundle By Name(w751) -> ("Method.Lenses"=w750:T5[])
                n530 = In Range and Coerce(upper limit=1000000, x="# of Cycles", lower limit=1) -> (coerced(x)=w745:i32)  [unwired: 1 out]
                n531 = local read "Mass Range"() -> (w742:i32)
                n532 = In Range and Coerce(upper limit=w740, x="Pause Time (ms)", lower limit=w741) -> (coerced(x)=w746:dbl)  [unwired: 1 out]
                n533 = In Range and Coerce(upper limit=w740, x="Delay Time (ms)", lower limit=w741) -> (coerced(x)=w739:dbl)  [unwired: 1 out]
                n534 = Index Array(array=w750, index=w749) -> (element=w752:T5)
                n535 = Bundle By Name(cluster=w752, "Scans"=w745, "Time 2"=w746, "Time 1"=w739) -> (w748:T5)
                n536 = property on="Mass Range" class="MCListbox (strict)"("Val(Sgnl)"=w742) -> ()  [unwired: 2 in, 2 out]
                n537 = Replace Array Subset(array=w750, new element=w748, index=w749) -> (w747:T5[])
                n538 = Bundle By Name(cluster=w751, "Method.Lenses"=w747) -> (w744:T20)
              }
              event "Start Mass (amu)", "Stop Mass (amu)", "Dwell Time (ms)", "Step Mass (amu)": Value Change {
                n539 = event-data() -> ()  [unwired: 7 out]
                n540 = Unbundle By Name(w773) -> ("Method.Mass Ranges"=w775:T6[])
                n541 = local read "Mass Range"() -> (w774:i32)
                n542 = local read "Center/Width"() -> (w757:bool)
                n543 = local read "Scan Type"() -> (w758:T2)
                n544 = property on="Mass Range" class="MCListbox (strict)"("Val(Sgnl)"=w774) -> ()  [unwired: 2 in, 2 out]
                n545 = Index Array(array=w775, index=w774) -> (element=w769:T6)
                n546 = Unbundle By Name(w769) -> ("Step Size"=w767:dbl)
                n547 = Not Equal?(x="Step Mass (amu)", y=w767) -> (x != y?=w760:bool)
                n548 = call "_Convert Center Width.vi"("Center/Width"=w757, "Run Mode"=w758, "StepMass Changed"=w760, "Step Mass"="Step Mass (amu)", "Stop Mass"="Stop Mass (amu)", "Start Mass"="Start Mass (amu)") -> ("Step Mass (amu)"=w763:dbl, "Stop Mass (amu)"=w762:dbl, "Start Mass (amu)"=w761:dbl)  [unwired: 1 out]
                n549 = Bundle By Name(cluster=w769, "Dwell"="Dwell Time (ms)", "Start"=w761, "Stop"=w762, "Step Size"=w763, "Res"="Resolution (Q1/Q2)") -> (w768:T6)
                n550 = Replace Array Subset(array=w775, new element=w768, index=w774) -> (w772:T6[])
                n551 = Bundle By Name(cluster=w773, "Method.Mass Ranges"=w772) -> (w771:T20)
              }
              event "Insert Row": Value Change {
                n552 = event-data() -> ()  [unwired: 7 out]
                n553 = Unbundle By Name(w777) -> ("Method.Mass Ranges"=w781:T6[])
                n554 = local read "Mass Range"() -> (w780:i32)
                n555 = property on="Mass Range" class="MCListbox (strict)"("Val(Sgnl)"=w780) -> ()  [unwired: 2 in, 2 out]
                n556 = Index Array(array=w781, index=w780) -> (element=w779:T6)
                n557 = Insert Into Array(array=w781, index=w780, new element=w779) -> (w778:T6[])
                n558 = Bundle By Name(cluster=w777, "Method.Mass Ranges"=w778) -> (w776:T20)
              }
              event "Delete Row": Value Change {
                n559 = event-data() -> ()  [unwired: 7 out]
                n560 = Unbundle By Name(w784) -> ("Method.Mass Ranges"=w783:T6[])
                n561 = Array Size(array=w783) -> (size(s)=w786:i32)
                n562 = Greater?(x=w786, y=1) -> (0:w785:bool)
                n563 = case shown="True" w785 {
                  tunnel: w784 -> [w788 w792]
                  tunnel: w783 -> [_ w794]
                  tunnel: [w788 w790] -> w782
                  frame False {
                    n564 = One Button Dialog(message="You are not allowed to delete the last mass range entry.") -> ()  [unwired: 2 out]
                  }
                  frame True {
                    n565 = local read "Mass Range"() -> (w793:i32)
                    n566 = property on="Mass Range" class="MCListbox (strict)"("Val(Sgnl)"=w793) -> ()  [unwired: 2 in, 2 out]
                    n567 = Delete From Array(array=w794, length=1, index=w793) -> (array with subset deleted=w791:T6[])  [unwired: 1 out]
                    n568 = Bundle By Name(cluster=w792, "Method.Mass Ranges"=w791) -> (w790:T20)
                  }
                }
              }
              event "MR Parameters": Value Change {
                n569 = event-data() -> ()  [unwired: 7 out]
                n570 = Unbundle By Name(w801) -> ("Method.Mass Ranges"=w799:T6[])
                n571 = local read "Mass Range"() -> (w800:i32)
                n572 = call "Mass Dependent Parameters.vi"("Current Mass Range"=w800, "Mass Ranges"=w799) -> ("Mass Ranges Out"=w798:T6[])  [unwired: 5 out]
                n573 = Bundle By Name(cluster=w801, "Method.Mass Ranges"=w798) -> (w796:T20)
                n574 = Unbundle By Name(w796) -> ("Method"=w797:T4)
                n575 = local write "Method"(w797) -> ()
              }
              event "CEM POL": Value Change {
                n576 = event-data() -> ("OldVal"=w802:bool)  [unwired: 6 out]
                n577 = Unbundle By Name(w804) -> ("Running"=w803:bool)
                n578 = case shown="False" w803 {
                  tunnel: w802 -> [_ w814]
                  frame False {
                    n579 = Number To Boolean Array(number=u16 0) -> (Boolean array=w811:bool[])
                    n580 = Replace Array Subset(array=w811, new element #1="CEM POL", index #1=0 ("index"), new element #2="CEM POL", index #2=1 ("index")) -> (w808:bool[])
                    n581 = Boolean Array To Number(Boolean array=w808) -> (number=w806:u16)
                    n582 = call "_Remote Communicate.vi"("DC Param"=w806, "Command"=_RT_Command."P3") -> ()  [unwired: 4 in, 4 out]
                  }
                  frame True {
                    n583 = local write "CEM POL"(w814) -> ()
                    n584 = One Button Dialog(message="Cannot change CEM polarity during a run") -> ()  [unwired: 2 out]
                  }
                }
              }
              event "Perform Parameter Ramp", "Start Value", "Stop Value", "Step Value", "Ramping Parameter": Value Change {
                n585 = event-data() -> ()  [unwired: 2 out]
                n586 = property on="Ramping Parameter" class="Ring (strict)"() -> ("Strings []"=w832:string[])  [unwired: 2 in, 2 out]
                n587 = Index Array(array=w832, index="Ramping Parameter") -> (element=w831:string)
                n588 = call "_Get Lens Configuration.vi"("Name"=w831) -> ("Lens Configuration"=w830:T19)  [unwired: 1 in, 5 out]
                n589 = Unbundle By Name(w830) -> ("Name"=w829:string, "Ch#"=w828:u8, "Min"=w822:dbl, "Max"=w823:dbl)
                n590 = In Range and Coerce(upper limit=w823, x="Start Value", lower limit=w822) -> (coerced(x)=w817:dbl)  [unwired: 1 out]
                n591 = In Range and Coerce(upper limit=w823, x="Stop Value", lower limit=w822) -> (coerced(x)=w816:dbl)  [unwired: 1 out]
                n592 = In Range and Coerce(upper limit=100.0, x="Step Value", lower limit=0.001) -> (coerced(x)=w815:dbl)  [unwired: 1 out]
                n593 = Select(t=w828, s="Perform Parameter Ramp", f=u8 0) -> (s? t:f=w826:u8)
                n594 = Bundle By Name(cluster=T7 {"Name"="", "Ch#"=0, "StartV"=0.0, "StopV"=100.0, "StepV"=1.0, "Index"=0} ("MR Parameters"), "Name"=w829, "Ch#"=w826, "Index"="Ramping Parameter", "StartV"=w817, "StopV"=w816, "StepV"=w815) -> (w833:T7)
                n595 = local write "Stop Value"(w816) -> ()
                n596 = local write "Start Value"(w817) -> ()
                n597 = local write "Step Value"(w815) -> ()
                n598 = global write "_Global Configuration.vi" "Scan Ramp"(w833) -> ()
              }
            }
          }
        }
        frame #2 {
          n599 = property class="VI"(reference=w838, error in=w837, "Front Panel Window:Open"=TRUE) -> (reference out=w841:refnum<vi>, error out=w840:errorcluster)
          n600 = Close Reference(reference=w842) -> ()  [unwired: 1 in, 1 out]
          n601 = Release Queue(queue=w843) -> ()  [unwired: 1 in, 4 out]
          n602 = Close Reference(reference=w841, error in (no error)=w840) -> ()  [unwired: 1 out]
        }
      }
    }
  }
